vi "DSPS_E36000.Manager.vi"(11 "Module Config":T2={"Name"="Serial Port", "Parent Q"=refnum, "Is Child?"=FALSE, "Index"=0, "Dirs"={"Root"=path "", "Config"=path "C:/ATE/Config", "Logs"=path "C:/ATE/Logs", "Reports"=path "C:/ATE/Reports", "App Data"=path "C:/ProgramData/MAIN"}, "Simulate"=FALSE, "SimCtrl"=refnum}) -> ()   [LabVIEW 2018]
uses:
  <vilib>/KATE/Module/Module Config.ctl
  <vilib>/KATE/Queues/Q.Element.ctl
  <vilib>/KATE/Module/Module.Working Dirs.ctl
  <vilib>/KATE/Event Log/Event Notification/Event Log.Log Level.ctl
  <vilib>/KATE/Module/Module.SW Version Info.ctl
  <vilib>/KATE/Module/Window/Window.Task, Action.ctl
  Utils/Functions/FunctMgr/FunctMgr.lvclass
  Utils/Errors/Error.Error Code List.ctl
  <vilib>/Utility/sysdir.llb/System Directory Type.ctl
  <vilib>/KATE/Event Log/Event Notification/Event Log.Notification Type.ctl
  <vilib>/KATE/Config/Stored Controls/Class.SaveCtrls.lvclass
  <vilib>/KATE/Queues/Queue Utils.lvlib
  <vilib>/KATE/Module/Module Utils.lvlib
  <vilib>/KATE/Event Log/Event Log.lvlib
  <vilib>/KATE/Scheduler/Scheduler.lvlib
  <vilib>/KATE/Menu/Menu Utils.lvlib
  <vilib>/KATE/Config/Config Utils.lvlib
  <vilib>/KATE/Status/Status Utils.lvlib
  <vilib>/KATE/Files/File Utils.lvlib
  <vilib>/KATE/SeqMgr/SeqMgr.lvlib
  <vilib>/KATE/Event Log/Event Notification/Event Notification.lvclass
panel:
  in  "Main Tab":enum32{"Operate", "Maint"}(tab)
  in  "Data Tab":enum32{"Control", "Config"}(tab)
  in  "Save Current to File":bool
  out "PS Output State":bool
  in  "Interval(s)":dbl=0.1 min=0.1 max=10.0 step=0.1
  in  "Continuous Read":bool
  in  "Current Lim":dbl=1.0
  in  "PS - Set Output OFF":bool
  in  "Voltage":dbl=12.0
  out "Current(A)":dbl format="%#.3f"
  in  "Read Current":bool
  in  "PS - Set Output ON":bool
  in  "Alias":refnum<visa-resource-name>="PS1"
  out "Status":string
  out "Current Graph":cluster{"t":dbl[], "Y":dbl[]}(graph)
  in  "Clear Current Graph":bool
  out "CurrAvg(A)":dbl caption="Average(A)" format="%#.3f"
  out "CurrPeak(A)":dbl caption="Peak(A)" format="%#.3f"
  in  "Average Cnt":i32=1 caption="Average Samples" min=1 max=100 step=1
  in  "Toggle Sim":bool
  in  "Get ID":bool
  out "FW":string
  out "SN":string
  out "Model":string
  out "Mfg":string
  out "Error":errorcluster
  in  "Logging Level":T1
  out "Rev":string="v1.0.0"
  out "Simulate Indication":string="Simulating Instruments"
  out "Error Status":string
  in  "Clear Error":bool
  in  "Leave Maint":bool
  # "Power Supply Manager"
  # "Output"
  # "V"
  # "A"
  # "Current"
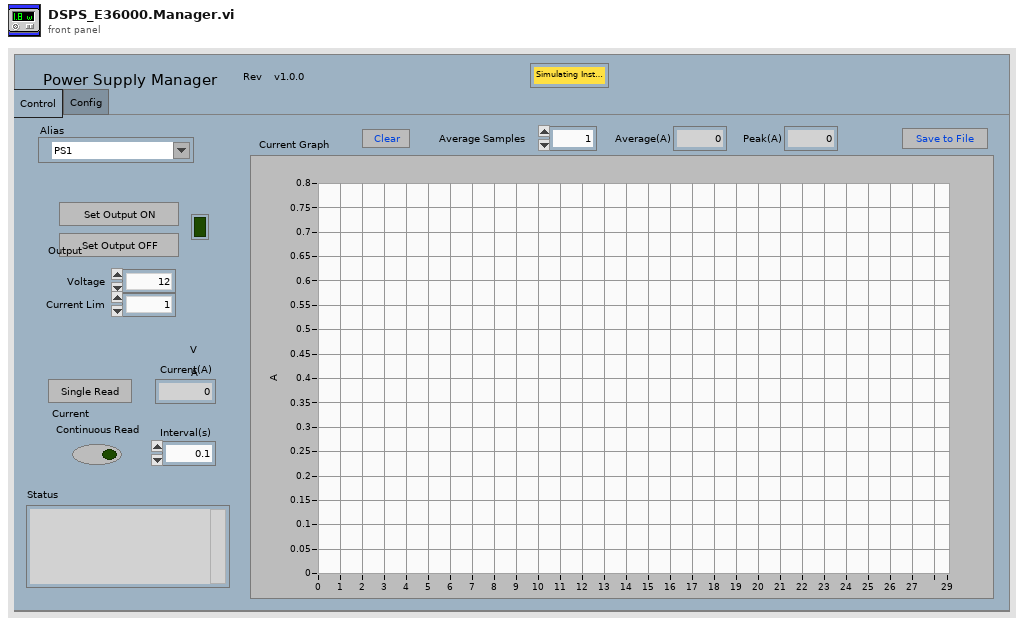
[diagram p1: front panel]
types:
  T1 = typedef "KATE_Lib.lvlib/Event Log.lvlib/Event Log.Log Level.ctl" = enum16{"Normal", "Verbose", "Debug0", "Debug1", "Debug2"}
  T2 = typedef "KATE_Lib.lvlib/Module Utils.lvlib/Module Config.ctl" = cluster{"Name":string, "Parent Q":refnum<queue>, "Is Child?":bool, "Index":i32, "Dirs":T3, "Simulate":bool, "SimCtrl":refnum<vi>}
  T3 = typedef "KATE_Lib.lvlib/Module Utils.lvlib/Module.Working Dirs.ctl" = cluster{"Root":path, "Config":path, "Logs":path, "Reports":path, "App Data":path}
  T4 = typedef "KATE_Lib.lvlib/Module Utils.lvlib/Module.SW Version Info.ctl" = cluster{"AppName":string, "Company":string, "Version":string, "Description":string, "PN":string}
  T5 = typedef "KATE_Lib.lvlib/Module Utils.lvlib/Module Sys Info.ctl" = cluster{"Main Q":refnum<queue>, "Exe":bool, "SW Rev":T4, "Self Ref":refnum<vi>, "Main Tab":refnum<vi>, "Pane":refnum<vi>, "Stop":cluster{"Ref":refnum<event-registration>, "Event":refnum<user-event>}, "Cfg":T2, "Services":cluster{"Name":string, "vi ref":refnum<vi>}[], "Menu Ref":refnum<k9>, "CtrlStates":refnum<class "Class.SaveCtrls.lvclass">, "Docs":cluster{"Tags":string[], "Paths":path[]}, "Log":refnum<class "Event Notification.lvclass">, "Test Controls":refnum<vi>[], "Child Modules":cluster{"Name":string, "vi ref":refnum<vi>}[], "SW Items":string[][], "AppData":refnum<class "Class.AppData.lvclass">}
  T6 = enum8{"Enabled", "Disabled", "Disabled and Grayed Out"}
  T7 = enum16{"open", "replace", "create", "open or create", "replace or create", "replace or create with confirmation"}
  T8 = typedef "KATE_Lib.lvlib/Event Log.lvlib/Event Log.Notification Type.ctl" = enum16{"Normal", "Warning", "Error", "Success"}
  T9 = cluster{"Child Modules":cluster{"VI Ref":refnum<vi>, "Name":string}[]}
  T10 = cluster{"Local Error":errorcluster, "Lnch":bool, "FunctMgr":refnum<class "FunctMgr.lvclass">, "App":cluster{"Child Modules":cluster{"VI Ref":refnum<vi>, "Name":string}[]}, "Alias":refnum<visa-resource-name>, "GraphData":cluster{"t":dbl[], "Y":dbl[]}, "Current":dbl, "GraphStart":dbl, "Connected":bool}
  T11 = typedef "Error.Error Code List.ctl" = i32
  T12 = typedef "System Directory Type.ctl" = i32
  T13 = typedef "KATE_Lib.lvlib/Module Utils.lvlib/Window.Task, Action.ctl" = enum16{"Resize()", "Show Panel(Bool)", "Show Scroll Bars(Bool)", "Dock to SubPanel(SubPanel Ref)", "Undock from SubPanel()", "Return to SubPanel()", "Go To Maint Tab()", "Show Maint Tab(Bool)", "Open Block Diagram()"}
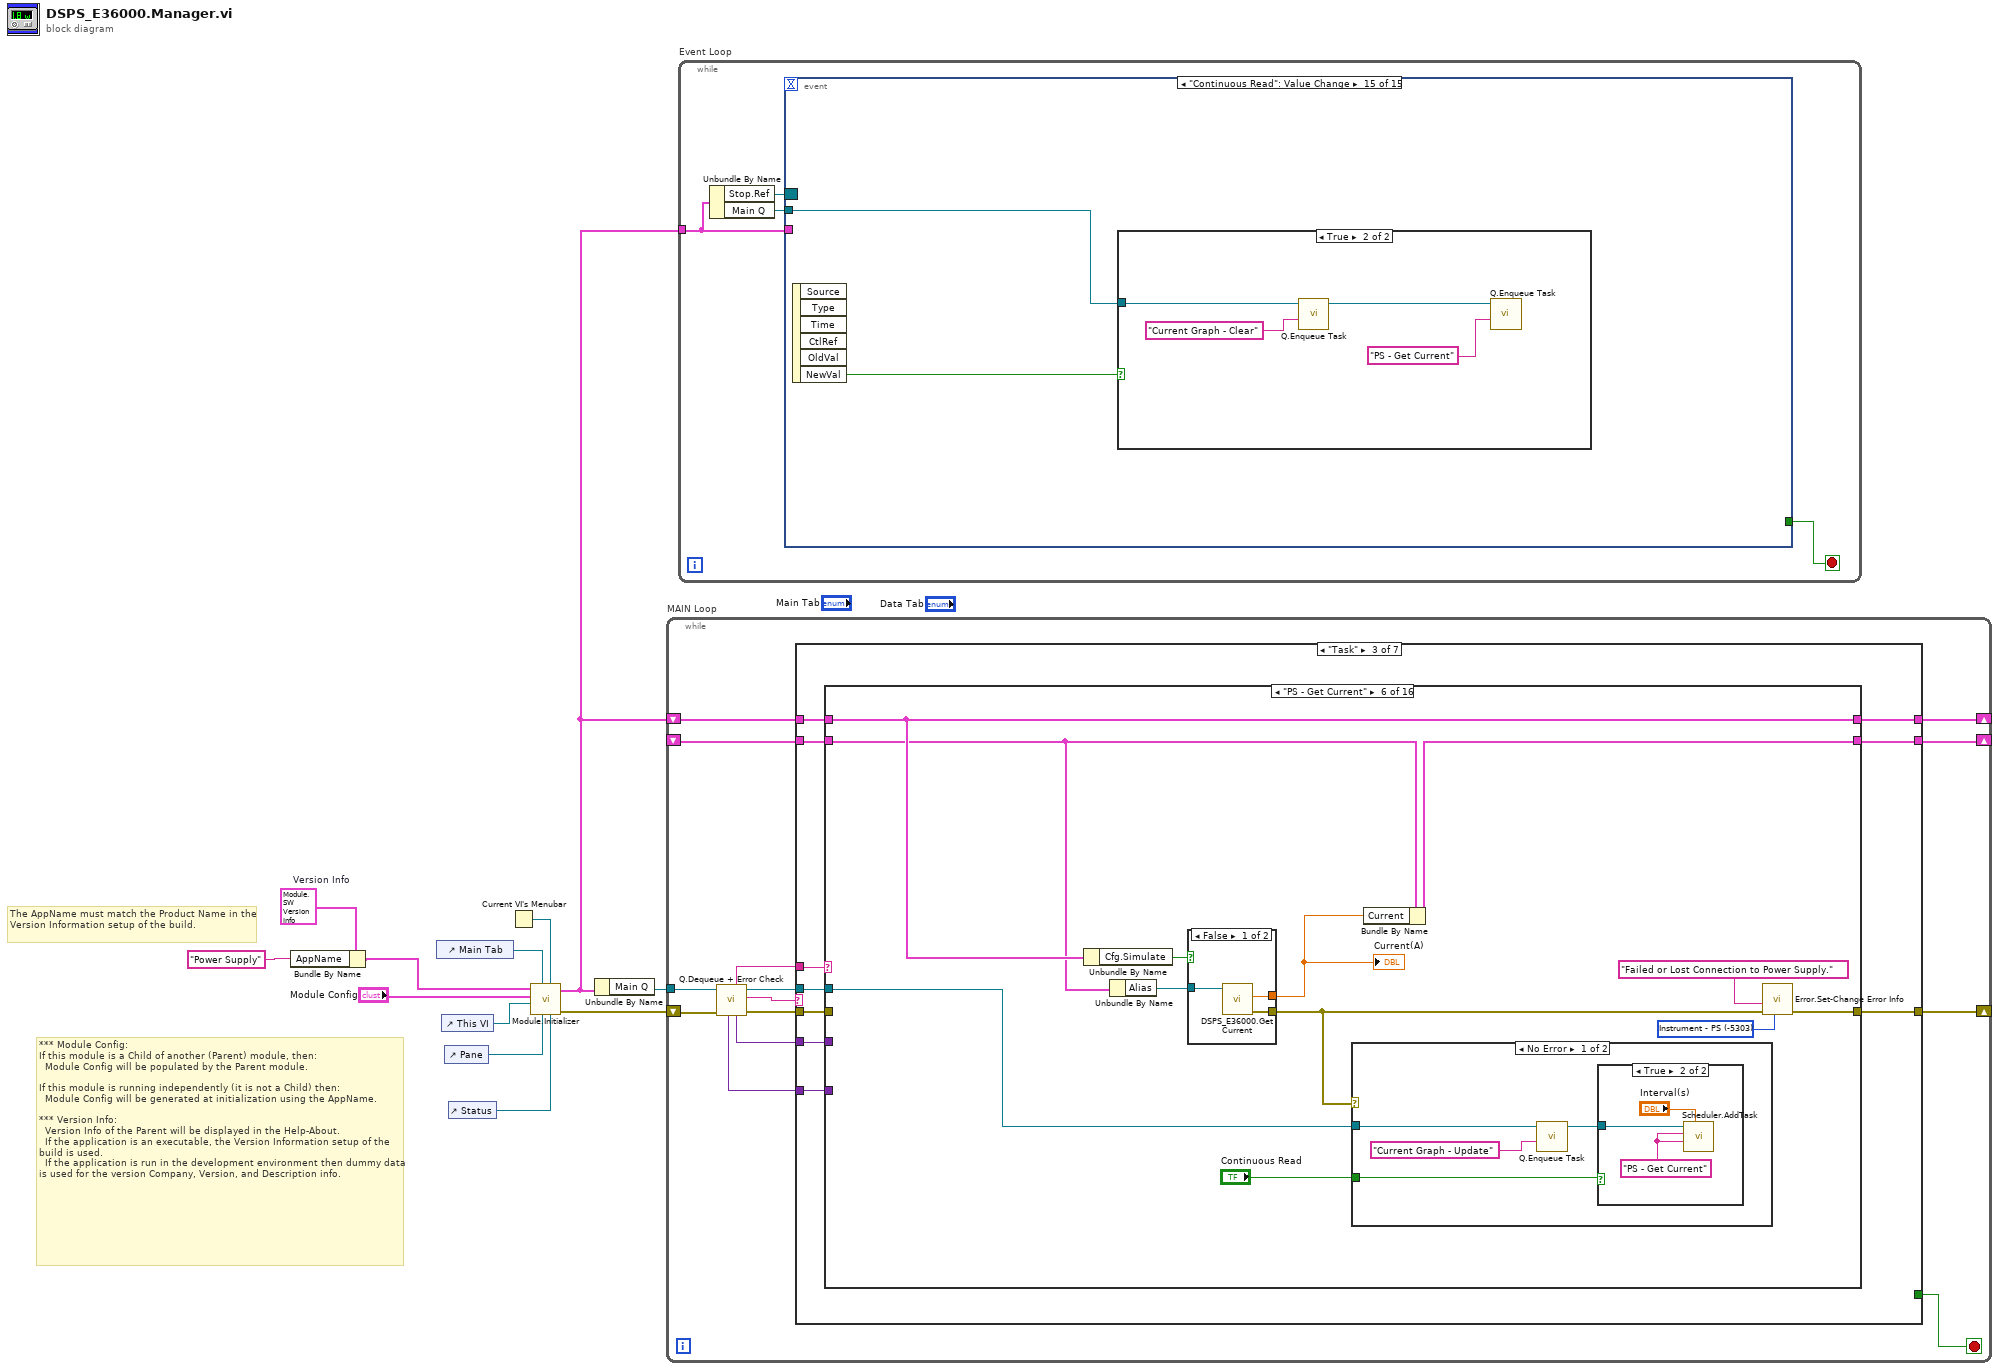
[diagram p0: block diagram]
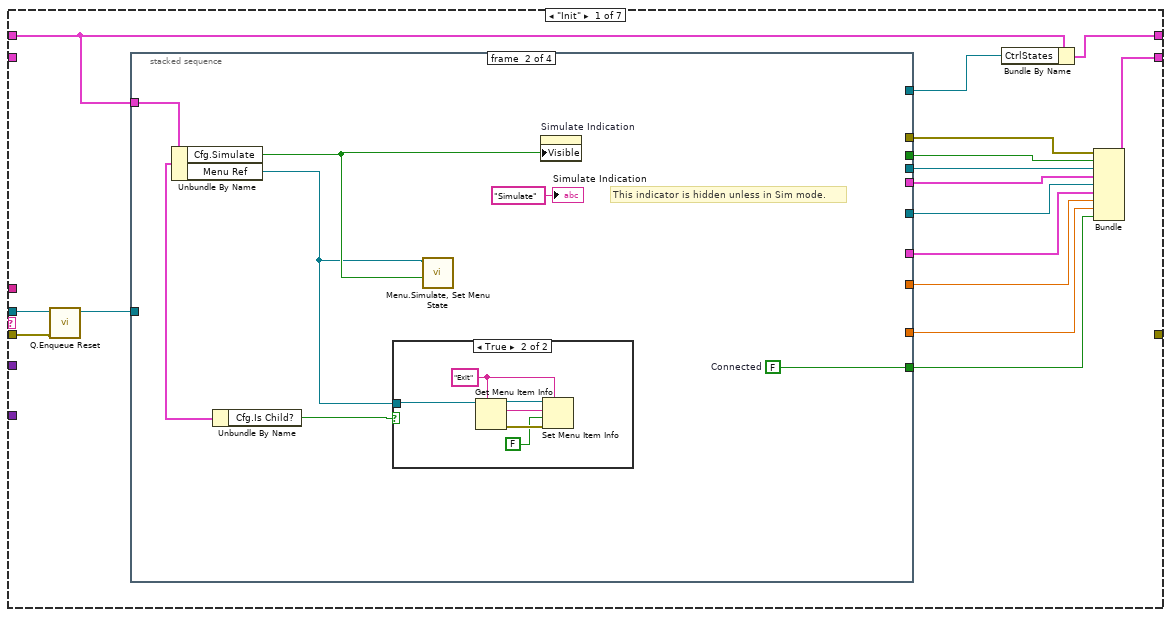
[diagram p2: hidden frame]
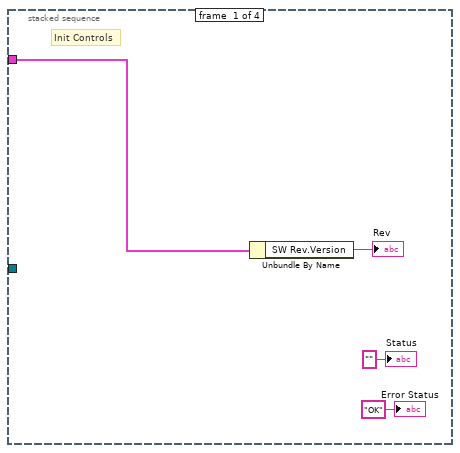
[diagram p3: hidden frame]
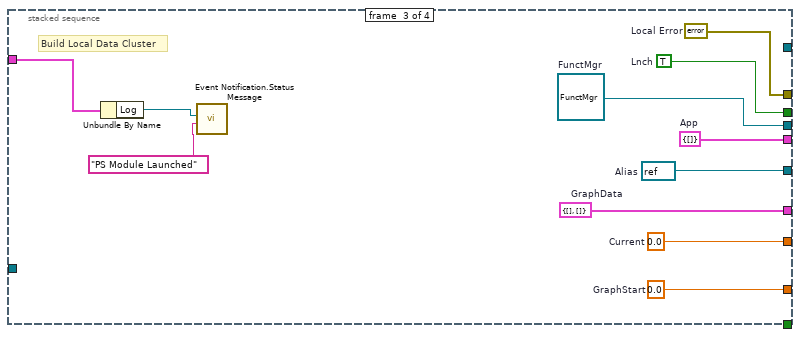
[diagram p5: hidden frame]
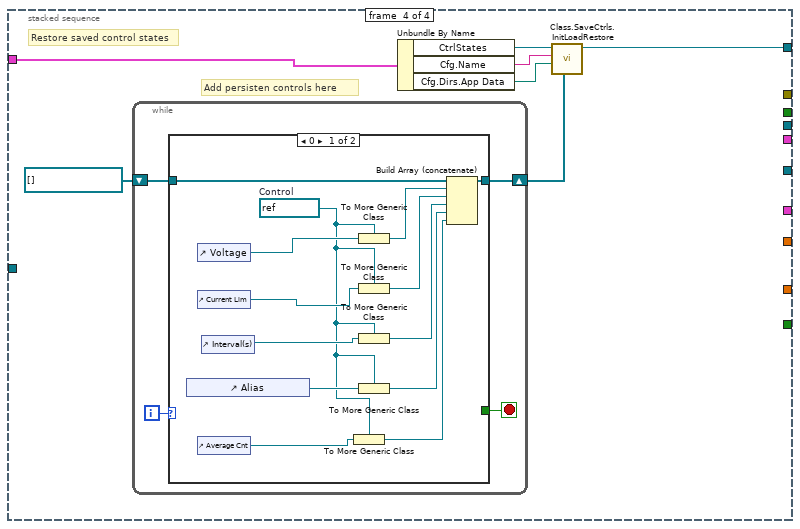
[diagram p6: hidden frame]
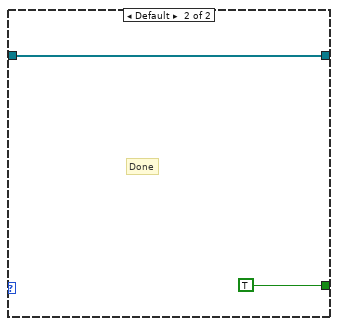
[diagram p7: hidden frame]
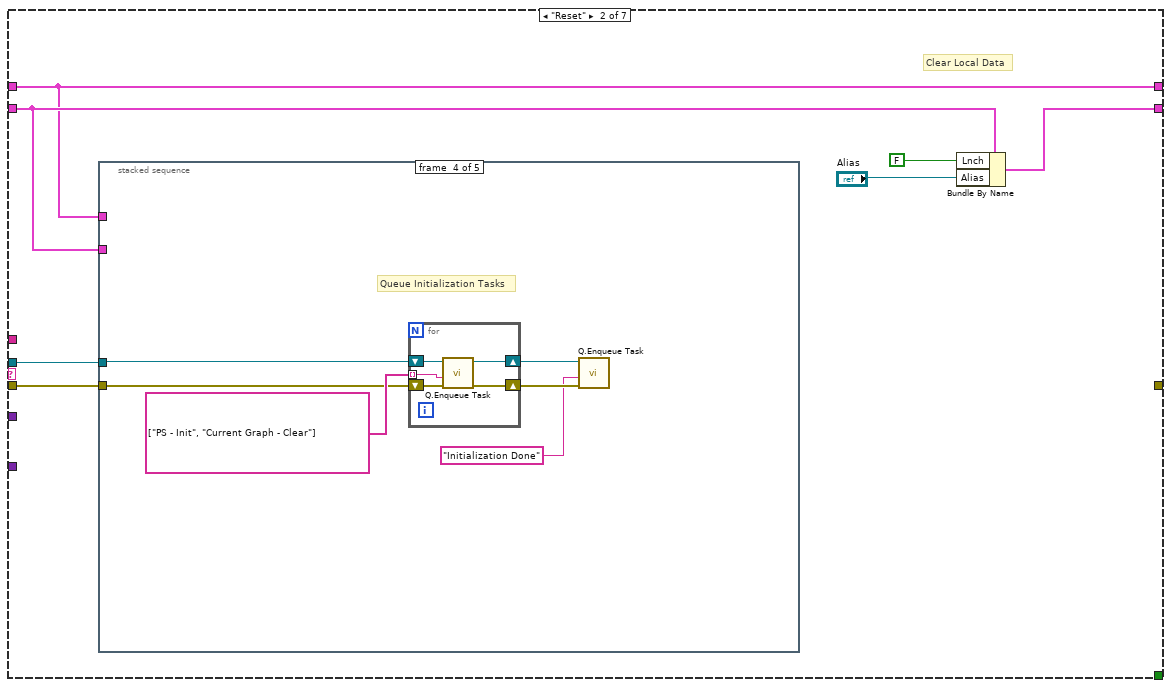
[diagram p8: hidden frame]
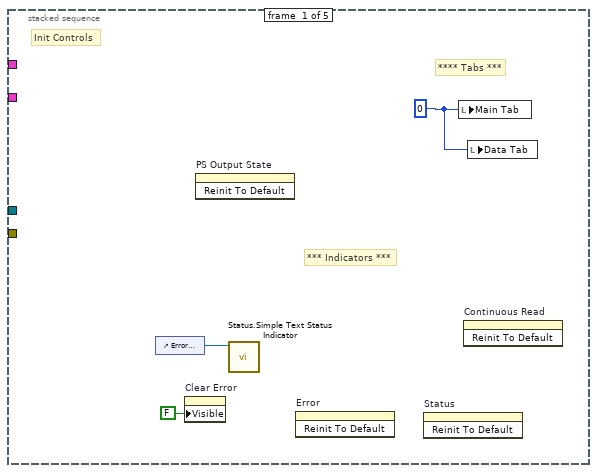
[diagram p9: hidden frame]
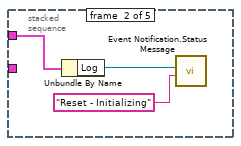
[diagram p10: hidden frame]
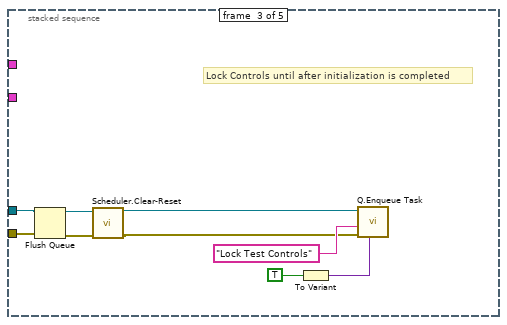
[diagram p11: hidden frame]
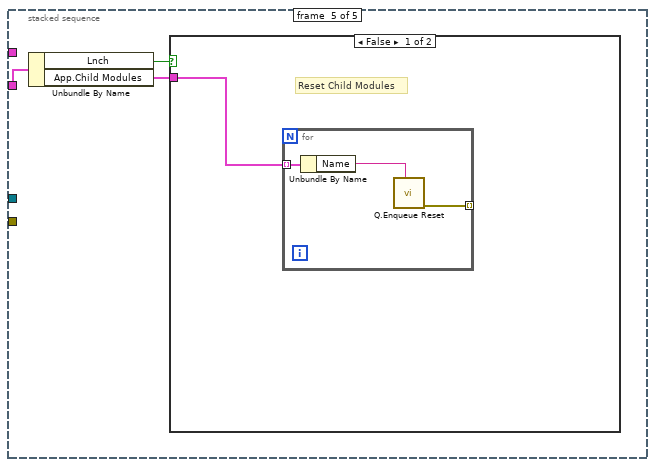
[diagram p12: hidden frame]
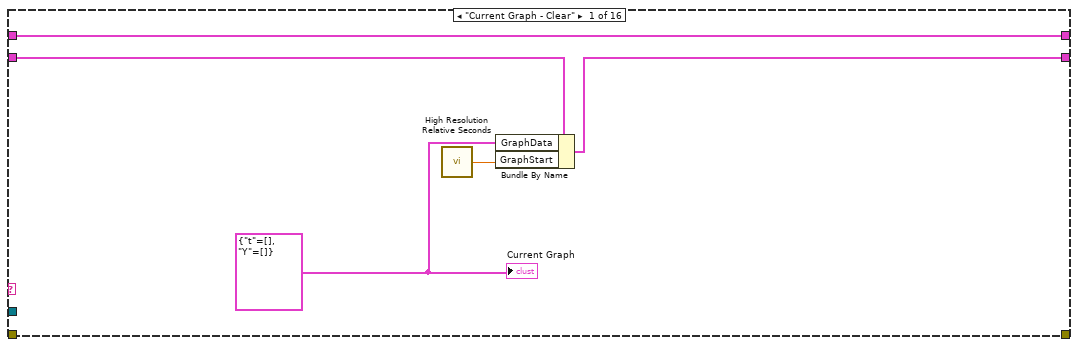
[diagram p14: hidden frame]
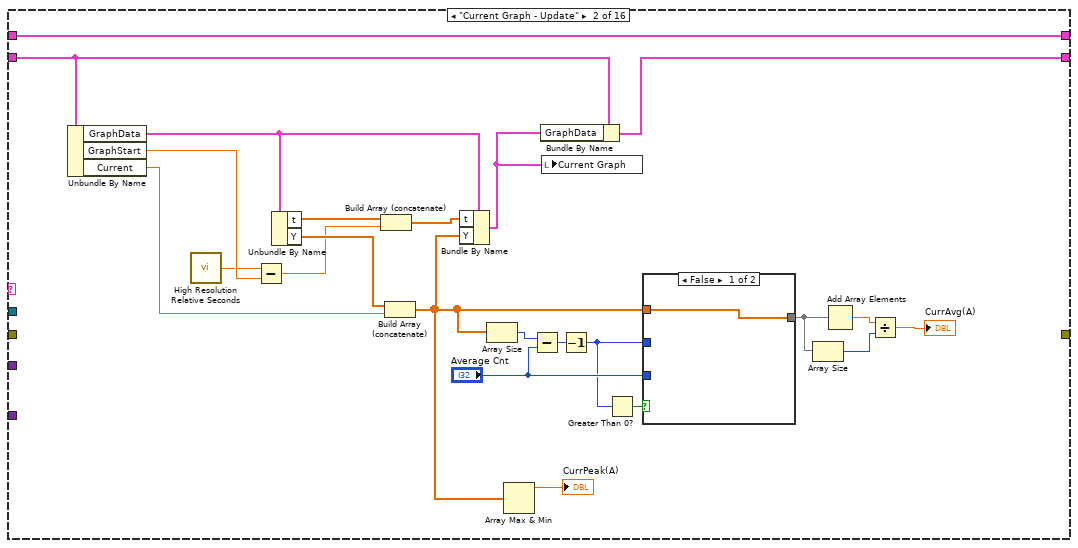
[diagram p15: hidden frame]
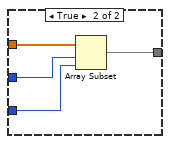
[diagram p16: hidden frame]
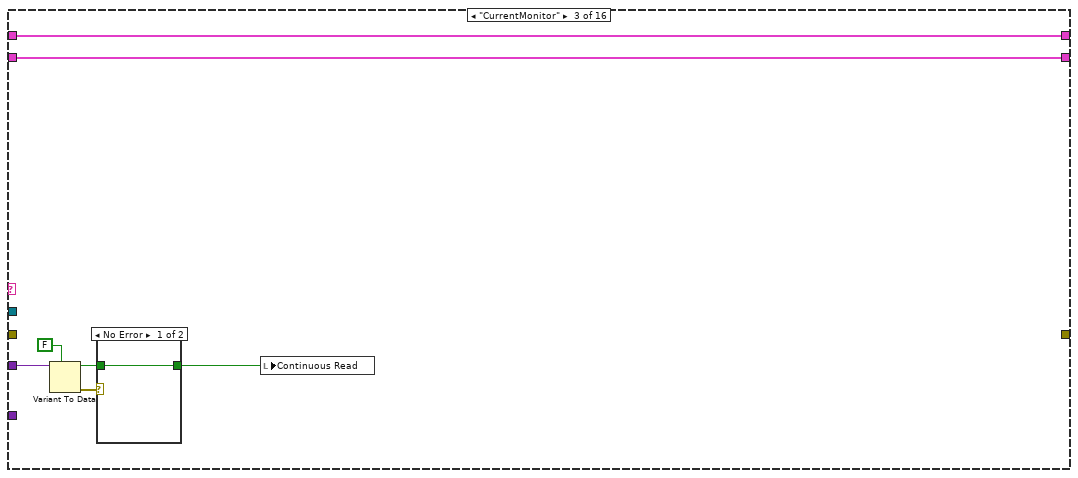
[diagram p17: hidden frame]
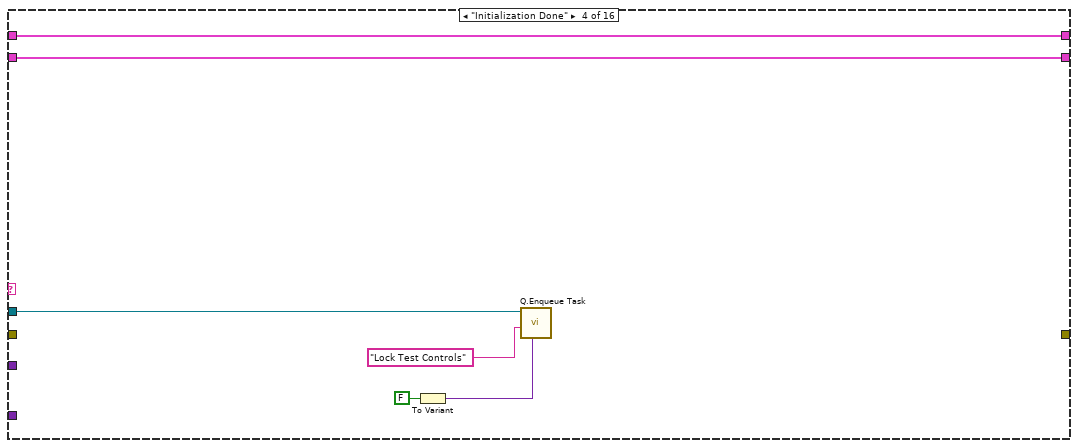
[diagram p19: hidden frame]
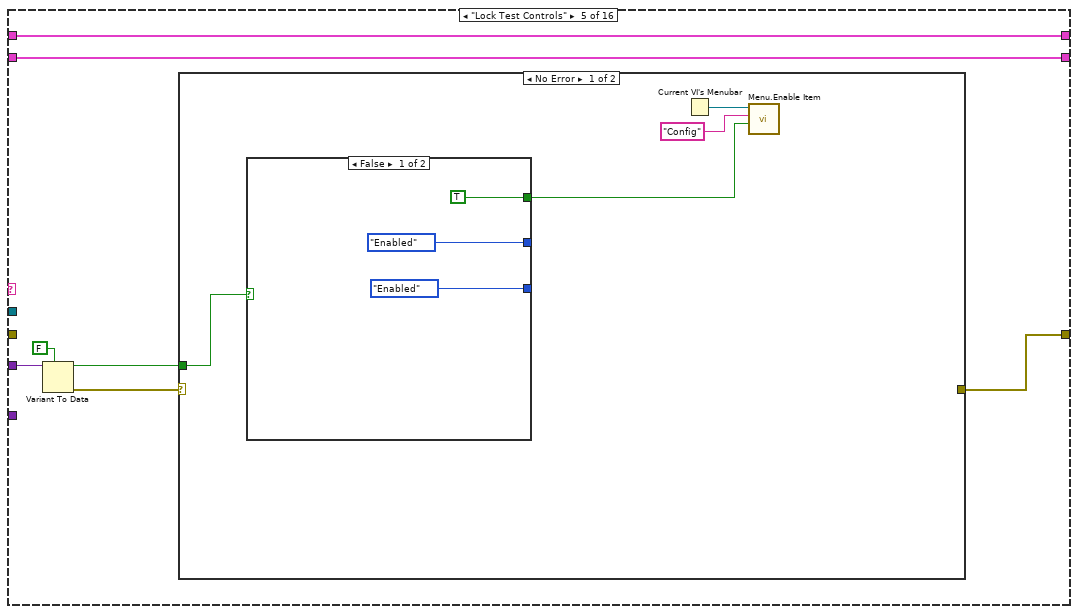
[diagram p20: hidden frame]
diagram:
  w2 = T4 {"AppName"="ModuleX", "Company"="CompanyX", "Version"="1.0", "Description"="This app is being developed.", "PN"=""}  # Version Info
  # "*** Module Config:\nIf this module is a Child of another (Parent) module, then:\n  Module Config will be populated by the Parent module.\n\nIf this module is running independently (it is not a Child) then:\n  Module Config will be generated at initialization using the AppName.\n\n*** Version Info:\n  Version Info of the Parent will be displayed in the Help-About.\n  If the application is an executable, the Version Information setup of the build is used.\n  If the application is run in the development environment then dummy data is used for the version Company, Version, and Description info."
  # "The AppName must match the Product Name in the Version Information setup of the build."
  n1 = Bundle By Name(cluster=w2, "AppName"="Power Supply") -> (w1:T4)
  n2 = control-ref of="Main Tab"() -> (w10:refnum<vi>)
  n3 = control-ref of="This VI"() -> (w9:refnum<vi>)
  n4 = control-ref of="Pane"() -> (w8:refnum<vi>)
  n5 = control-ref of="Status"() -> (w4:refnum<vi>)
  n6 = Current VI's Menubar() -> (w6:refnum<k9>)
  n7 = call <vilib>:"Module.Initializer.vi"("StatusTxtBx"=w4, "Menu Ref"=w6, "Pane"=w8, "Main Tab"=w10, "Self Ref"=w9, "Module Config"="Module Config", "SW Rev"=w1) -> ("error out"=w12:errorcluster, "Sys"=w7:T5)  [unwired: 3 in]
  n8 = Unbundle By Name(w7) -> ("Main Q"=w11:refnum<queue>)
  n9 = while "MAIN Loop" {
    shift-right: [w23] -> _
    shift-left: w12 -> [w21]
    shift-right: [w24] -> _
    shift-left: _ -> [w13]
    shift-right: [w25] -> _
    shift-left: w7 -> [w26]
    tunnel: w11 -> [w20]
    stop <- w15 stop-if-true
    n10 = call <vilib>:"Q.Dequeue + Error Check.vi"("Error In"=w21, "Q In"=w20) -> ("error out"=w22:errorcluster, "Cmd"=w19:string, "Q Out"=w18:refnum<queue>, "Data1"=w17:variant, "Sub"=w14:string, "Data2"=w16:variant)  [unwired: 4 in]
    n11 = case shown="\"Task\"" w19 {
      selector: w19 -> [_ _ _ _ _ w612 _]
      tunnel: w13 -> [_ w99 w144 w407 w586 w606 w671]
      tunnel: w26 -> [w37 w97 w145 w408 w587 w607 w672]
      tunnel: [w38 w97 w143 w406 w585 w607 w672] -> w25
      tunnel: [w40 w102 w142 w405 w584 w605 w671] -> w24
      tunnel: [_ _ w136 w400 _ w613 w674] -> w23
      tunnel: w22 -> [w41 w100 w138 w401 _ w610 _]
      tunnel: w18 -> [w42 w101 w139 w402 w590 w608 _]
      tunnel: w17 -> [_ _ w140 w403 w589 w611 _]
      tunnel: w16 -> [_ _ w137 w399 w588 _ _]
      tunnel: w14 -> [_ _ w141 w404 w591 w609 _]
      tunnel: [_ _ _ _ _ _ TRUE] -> w15
      frame "Init" {
        n12 = call <vilib>:"Q.Enqueue Reset.vi"("Error In"=w41, "Q In"=w42) -> ("Q Out"=w35:refnum<queue>)  [unwired: 8 in, 1 out]
        n13 = stacked-sequence {
          tunnel: [_ _ w63 _] -> w39
          tunnel: w37 -> [w45 w49 w66 w71]
          tunnel: [_ _ _ w70] -> w36
          tunnel: w35 -> [_ _ _ _]
          tunnel: [_ _ w69 _] -> w34
          tunnel: [_ _ w68 _] -> w33
          tunnel: [_ _ w61 _] -> w32
          tunnel: [_ _ w67 _] -> w31
          tunnel: [_ _ w62 _] -> w30
          tunnel: [_ _ w60 _] -> w29
          tunnel: [_ _ w59 _] -> w28
          tunnel: [_ w47 _ _] -> w27
          frame #0 {
            # "Init Controls"
            n14 = Unbundle By Name(w45) -> ("SW Rev.Version"=→"Rev":string)
            "Status" <- "" ("Status")
            "Error Status" <- "OK" ("Error Status")
          }
          frame #1 {
            w47 = FALSE  # Connected
            # "This indicator is hidden unless in Sim mode."
            n15 = Unbundle By Name(w49) -> ("Cfg.Simulate"=w51:bool, "Menu Ref"=w48:refnum<k9>)
            n16 = Unbundle By Name(w49) -> ("Cfg.Is Child?"=w50:bool)
            n17 = case shown="True" w50 {
              tunnel: w48 -> [_ w54]
              frame False {
              }
              frame True {
                w56 = "Exit"
                n18 = Get Menu Item Info(7:w56, 11:w54) -> (0:w55:errorcluster, 2:w57:string, 3:w58:refnum<k9>)  [unwired: 1 in, 4 out]
                n19 = Set Menu Item Info(7:w56, 8:w55, 9:FALSE ("enabled"), 10:w57, 11:w58) -> ()  [unwired: 2 in, 2 out]
              }
            }
            n20 = call <vilib>:"Menu.Simulate, Set Menu State.vi"("Sim Enable"=w51, "Menu Ref"=w48) -> ()  [unwired: 8 in, 2 out]
            n21 = property on="Simulate Indication" class="Str"("Visible"=w51) -> ()  [unwired: 2 in, 2 out]
            "Simulate Indication" <- "Simulate" ("Simulate Indication")
          }
          frame #2 {
            w59 = 0.0  # GraphStart
            w60 = 0.0  # Current
            w61 = refnum<visa-resource-name> refnum  # Alias
            w62 = cluster{"t":dbl[], "Y":dbl[]} {"t"=[], "Y"=[]}  # GraphData
            w67 = errorcluster {"status"=FALSE, "code"=0, "source"=""}  # Local Error
            w63 = refnum<class "FunctMgr.lvclass"> refnum  # FunctMgr
            w68 = T9 {"Child Modules"=[]}  # App
            w69 = TRUE  # Lnch
            # "Build Local Data Cluster"
            n22 = Unbundle By Name(w66) -> ("Log"=w65:refnum<class "Event Notification.lvclass">)
            n23 = call <vilib>:"Event Notification.Status Message.vi"("Message"="PS Module Launched", "Event Notification in"=w65) -> ()  [unwired: 10 in]
          }
          frame #3 {
            # "Add persisten controls here"
            # "Restore saved control states"
            n24 = while {
              shift-right: [w78] -> w72
              shift-left: refnum<vi>[] [] -> [w79]
              i -> [w80]
              stop <- w77 stop-if-true
              n25 = case shown="0" w80 {
                tunnel: w79 -> [w92 w95]
                tunnel: [w93 w95] -> w78
                tunnel: [_ TRUE] -> w77
                frame 0 {
                  w83 = refnum<vi> refnum  # Control
                  n26 = control-ref of="Alias"() -> (w87:refnum<vi>)
                  n27 = control-ref of="Voltage"() -> (w84:refnum<vi>)
                  n28 = control-ref of="Current Lim"() -> (w85:refnum<vi>)
                  n29 = control-ref of="Average Cnt"() -> (w81:refnum<vi>)
                  n30 = control-ref of="Interval(s)"() -> (w86:refnum<vi>)
                  n31 = To More Generic Class(target class=w83, reference=w81) -> (generic class reference=w82:refnum<vi>)
                  n32 = To More Generic Class(target class=w83, reference=w84) -> (generic class reference=w91:refnum<vi>)
                  n33 = To More Generic Class(target class=w83, reference=w85) -> (generic class reference=w90:refnum<vi>)
                  n34 = To More Generic Class(target class=w83, reference=w86) -> (generic class reference=w89:refnum<vi>)
                  n35 = To More Generic Class(target class=w83, reference=w87) -> (generic class reference=w88:refnum<vi>)
                  n36 = Build Array (concatenate)(w92, w91, w90, w89, w88, w82) -> (w93:refnum<vi>[])
                }
                frame Default {
                  # "Done"
                }
              }
            }
            n37 = Unbundle By Name(w71) -> ("CtrlStates"=w73:refnum<class "Class.SaveCtrls.lvclass">, "Cfg.Name"=w75:string, "Cfg.Dirs.App Data"=w74:path)
            n38 = call-dynamic "Class.SaveCtrls.InitLoadRestore.vi"("Ctrl Array"=w72, "Module Data Dir"=w74, "Module Name"=w75, "CtrlStates In"=w73) -> ("CtrlStates"=w70:refnum<class "Class.SaveCtrls.lvclass">)  [unwired: 6 in, 1 out]
          }
        }
        n39 = Bundle By Name(cluster=w37, "CtrlStates"=w36) -> (w38:T5)
        n40 = Bundle("Local Error"=w31, "Lnch"=w34, "FunctMgr"=w39, "App"=w33, "Alias"=w32, "GraphData"=w30, "Current"=w29, "GraphStart"=w28, "Connected"=w27) -> (w40:T10)  [unwired: 1 in]
      }
      frame "Reset" {
        # "Clear Local Data"
        n41 = stacked-sequence {
          tunnel: w101 -> [_ _ w110 w118 _]
          tunnel: w100 -> [_ _ w109 w122 _]
          tunnel: w99 -> [_ _ _ _ w131]
          tunnel: w97 -> [_ w108 _ _ _]
          frame #0 {
            w105 = 0
            # "*** Indicators ***"
            # "**** Tabs ***"
            # "Init Controls"
            n42 = control-ref of="Error Status"() -> (w104:refnum<vi>)
            n43 = property on="Clear Error" class="Bool"("Visible"=FALSE) -> ()  [unwired: 2 in, 2 out]
            n44 = invoke on="PS Output State" class="Bool (strict)" method="Reinit To Default"() -> ()  [unwired: 3 in, 3 out]
            n45 = call <vilib>:"Status.Simple Text Status Indicator.vi"("Status TextBox"=w104) -> ()  [unwired: 10 in, 1 out]
            n46 = invoke on="Error" class="Clust (strict)" method="Reinit To Default"() -> ()  [unwired: 3 in, 3 out]
            n47 = invoke on="Status" class="Str" method="Reinit To Default"() -> ()  [unwired: 3 in, 3 out]
            n48 = local write "Main Tab"(w105) -> ()
            n49 = invoke on="Continuous Read" class="Bool (strict)" method="Reinit To Default"() -> ()  [unwired: 3 in, 3 out]
            n50 = local write "Data Tab"(w105) -> ()
          }
          frame #1 {
            n51 = Unbundle By Name(w108) -> ("Log"=w107:refnum<class "Event Notification.lvclass">)
            n52 = call <vilib>:"Event Notification.Status Message.vi"("Message"="Reset - Initializing", "Event Notification in"=w107) -> ()  [unwired: 10 in]
          }
          frame #2 {
            # "Lock Controls until after initialization is completed"
            n53 = Flush Queue(queue=w110, error in (no error)=w109) -> (queue out=w111:refnum<queue>, error out=w114:errorcluster)  [unwired: 1 out]
            n54 = call <vilib>:"Scheduler.Clear-Reset.vi"("error in"=w114, "Q In"=w111) -> ("error out"=w112:errorcluster, "Q Out"=w113:refnum<queue>)  [unwired: 8 in]
            n55 = To Variant(anything=TRUE) -> (Variant=w116:variant)
            n56 = call <vilib>:"Q.Enqueue Task.vi"("Data1"=w116, "Error In"=w112, "Task Name"="Lock Test Controls", "Q In"=w113) -> ()  [unwired: 6 in, 2 out]
          }
          frame #3 {
            # "Queue Initialization Tasks"
            n57 = for {
              shift-right: [w126] -> w120
              shift-left: w122 -> [w127]
              tunnel: string[] ["PS - Init", "Current Graph - Clear"] -> [w124] mode=indexing
              shift-right: [w125] -> w121
              shift-left: w118 -> [w128]
              n58 = call <vilib>:"Q.Enqueue Task.vi"("Error In"=w127, "Task Name"=w124, "Q In"=w128) -> ("error out"=w126:errorcluster, "Q Out"=w125:refnum<queue>)  [unwired: 7 in]
            }
            n59 = call <vilib>:"Q.Enqueue Task.vi"("Error In"=w120, "Task Name"="Initialization Done", "Q In"=w121) -> ()  [unwired: 7 in, 2 out]
          }
          frame #4 {
            n60 = Unbundle By Name(w131) -> ("Lnch"=w130:bool, "App.Child Modules"=w129:cluster{"VI Ref":refnum<vi>, "Name":string}[])
            n61 = case shown="False" w130 {
              tunnel: w129 -> [w132 _]
              frame False {
                # "Reset Child Modules"
                n62 = for {
                  tunnel: w132 -> [w135] mode=indexing
                  tunnel: [w133] -> _ mode=indexing
                  n63 = Unbundle By Name(w135) -> ("Name"=w134:string)
                  n64 = call <vilib>:"Q.Enqueue Reset.vi"("Q Name"=w134) -> ("error out"=w133:errorcluster)  [unwired: 9 in, 1 out]
                }
              }
              frame True {
                # "Do not reset at launch.\nThey are already reset"
              }
            }
          }
        }
        n65 = Bundle By Name(cluster=w99, "Lnch"=FALSE ("Test.Running"), "Alias"="Alias") -> (w102:T10)
      }
      frame "Task" {
        n66 = case shown="\"PS - Get Current\"" w141 {
          selector: w141 -> [_ _ _ _ _ _ _ _ _ _ _ _ _ _ _ w394]
          tunnel: w145 -> [w150 w173 w185 w192 w199 w220 w241 w265 w291 w309 w345 w351 w356 w372 w378 w389]
          tunnel: w144 -> [w149 w168 w184 w187 w193 w217 w247 w260 w293 w305 w344 w350 w360 w374 w377 w395]
          tunnel: [w150 w173 w185 w192 w199 w220 w241 w265 w291 w309 w345 w351 w361 w373 w378 w388] -> w143
          tunnel: [w148 w167 w184 w187 w193 w216 w247 w259 w293 w304 w344 w349 w360 w374 w377 w395] -> w142
          tunnel: w140 -> [_ _ w183 _ w198 _ _ _ w289 w301 _ _ w363 _ w379 w393]
          tunnel: w139 -> [_ _ _ w191 _ w221 _ w266 _ _ _ _ w357 w375 _ _]
          tunnel: w138 -> [_ _ _ _ _ _ _ _ _ _ _ _ _ _ _ w391]
          tunnel: w137 -> [_ _ _ _ _ _ _ _ _ w302 _ _ _ _ _ w392]
          tunnel: [_ _ _ _ w195 w212 w237 w256 w284 w303 _ _ _ _ w376 w390] -> w136
          frame "Current Graph - Clear" {
            w147 = cluster{"t":dbl[], "Y":dbl[]} {"t"=[], "Y"=[]}
            n67 = call <vilib>:"High Resolution Relative Seconds.vi"() -> ("relative seconds"=w146:dbl)
            n68 = Bundle By Name(cluster=w149, "GraphData"=w147, "GraphStart"=w146) -> (w148:T10)
            "Current Graph" <- w147
          }
          frame "Current Graph - Update" {
            n69 = Unbundle By Name(w168) -> ("GraphData"=w169:cluster{"t":dbl[], "Y":dbl[]}, "GraphStart"=w154:dbl, "Current"=w151:dbl)
            n70 = call <vilib>:"High Resolution Relative Seconds.vi"() -> ("relative seconds"=w153:dbl)
            n71 = Subtract(x=w153, y=w154) -> (x-y=w152:dbl)
            n72 = Unbundle By Name(w169) -> ("t"=w172:dbl[], "Y"=w170:dbl[])
            n73 = Build Array (concatenate)(w172, w152) -> (w171:dbl[])
            n74 = Build Array (concatenate)(w170, w151) -> (w165:dbl[])
            n75 = Bundle By Name(cluster=w169, "t"=w171, "Y"=w165) -> (w156:cluster{"t":dbl[], "Y":dbl[]})
            n76 = Array Size(array=w165) -> (size(s)=w164:i32)
            n77 = Array Max & Min(array=w165) -> (max value=→"CurrPeak(A)":dbl)  [unwired: 3 out]
            n78 = Subtract(x=w164, y="Average Cnt") -> (x-y=w163:i32)
            n79 = Bundle By Name(cluster=w168, "GraphData"=w156) -> (w167:T10)
            n80 = local write "Current Graph"(w156) -> ()
            n81 = Decrement(x=w163) -> (x-1=w160:i32)
            n82 = Greater Than 0?(x=w160) -> (x > 0?=w161:bool)
            n83 = case shown="False" w161 {
              tunnel: w165 -> [w174 w178]
              tunnel: w160 -> [_ w177]
              tunnel: "Average Cnt" -> [_ w176]
              tunnel: [w174 w175] -> w159
              frame False {
              }
              frame True {
                n84 = Array Subset(array=w178, index=w177, length=w176) -> (w175:dbl[])
              }
            }
            n85 = Array Size(array=w159) -> (size(s)=w157:i32)
            n86 = Add Array Elements(numeric array=w159) -> (sum=w158:dbl)
            n87 = Divide(x=w158, y=w157) -> (x/y=→"CurrAvg(A)":dbl)
          }
          frame "CurrentMonitor" {
            n88 = Variant To Data(type=FALSE, Variant=w183) -> (data=w180:bool, error out=w181:errorcluster)  [unwired: 1 in]
            n89 = case shown="No Error" w181 {
              tunnel: w180 -> [w186 _]
              tunnel: [w186 _] -> w179
              frame No Error {
              }
              frame Error {
              }
            }
            n90 = local write "Continuous Read"(w179) -> ()
          }
          frame "Initialization Done" {
            n91 = To Variant(anything=FALSE) -> (Variant=w189:variant)
            n92 = call <vilib>:"Q.Enqueue Task.vi"("Data1"=w189, "Task Name"="Lock Test Controls", "Q In"=w191) -> ()  [unwired: 7 in, 2 out]
          }
          frame "Lock Test Controls" {
            n93 = Variant To Data(type=FALSE, Variant=w198) -> (data=w194:bool, error out=w196:errorcluster)  [unwired: 1 in]
            n94 = case shown="No Error" w196 {
              selector: w196 -> [_ w210]
              tunnel: w194 -> [w203 _]
              tunnel: [_ w210] -> w195
              frame No Error {
                n95 = case shown="False" w203 {
                  tunnel: [T6."Enabled" ("Disabled") T6."Disabled and Grayed Out" ("Disabled")] -> _
                  tunnel: [T6."Enabled" ("Disabled") T6."Disabled" ("Disabled")] -> _
                  tunnel: [TRUE ("Enable") FALSE ("Enable")] -> w200
                  frame False {
                  }
                  frame True {
                  }
                }
                n96 = Current VI's Menubar() -> (w201:refnum<k9>)
                n97 = call <vilib>:"Menu.Enable Item.vi"("Enable"=w200, "Tag"="Config", "Menu Ref"=w201) -> ()  [unwired: 7 in, 2 out]
              }
              frame Error {
              }
            }
          }
          frame "PS - Get Current" {
            w214 = T11 -5303 items=["No Error"=0, "Abort"=-2, "Misc"=-5000, "Fixture Error"=-5100, "File IO - General"=-5200, "FIle IO - Config Error"=-5201, "Instrument - General"=-5300, "Instrument - Serial Com"=-5301, "Instrument - Camera"=-5302, "Instrument - PS"=-5303, "Instrument - Oscilloscope"=-5304, "Instrument - Function Gen"=-5305, "Instrument - Load"=-5306, "Instrument - Meter"=-5307, "Instrument - Power Control"=-5308, "Instrument - Motion"=-5309, "Instrument - RF"=-5310, "System Exe"=-5400, "Image Processing"=-5500, "Communication"=-5600, "Script - Syntax Error"=-6000, "Script - Invalid Name or Param"=-6100, "Script - Timeout"=-6200, "Invalid Data"=-6300] ("Std Code")
            n98 = Unbundle By Name(w220) -> ("Cfg.Simulate"=w219:bool)
            n99 = Unbundle By Name(w217) -> ("Alias"=w222:refnum<visa-resource-name>)
            n100 = case shown="False" w219 {
              tunnel: w222 -> [w225 _]
              tunnel: [w224 w228] -> w215
              tunnel: [w223 _] -> w211
              frame False {
                n101 = call "DSPS_E36000.Get Current.vi"("VISA Alias"=w225) -> ("error out"=w223:errorcluster, "Current"=w224:dbl)  [unwired: 7 in, 2 out]
              }
              frame True {
                n102 = Random Number (0-1)() -> (number: 0 to 1=w227:dbl)
                n103 = Multiply(x=w227, y=0.8) -> (x*y=w228:dbl)
              }
            }
            "Current(A)" <- w215
            n104 = case shown="No Error" w211 {
              tunnel: w221 -> [w231 _]
              tunnel: "Continuous Read" -> [w229 _]
              frame No Error {
                n105 = call <vilib>:"Q.Enqueue Task.vi"("Task Name"="Current Graph - Update" ("Name"), "Q In"=w231) -> ("Q Out"=w230:refnum<queue>)  [unwired: 8 in, 1 out]
                n106 = case shown="True" w229 {
                  tunnel: w230 -> [_ w235]
                  frame False {
                  }
                  frame True {
                    w234 = "PS - Get Current" ("Name")
                    n107 = call <vilib>:"Scheduler.AddTask.vi"("Interval(s)"="Interval(s)", "Task Name"=w234, "Sched Name"=w234, "Q In"=w235) -> ()  [unwired: 6 in, 2 out]
                  }
                }
              }
              frame Error {
              }
            }
            n108 = Bundle By Name(cluster=w217, "Current"=w215) -> (w216:T10)
            n109 = call "Error.Set-Change Error Info.vi"("Std Code"=w214, "error in"=w211, "Description"="Failed or Lost Connection to Power Supply.") -> ("error out"=w212:errorcluster)  [unwired: 8 in]
          }
          frame "PS - Get ID" {
            w239 = T11 -5303 items=["No Error"=0, "Abort"=-2, "Misc"=-5000, "Fixture Error"=-5100, "File IO - General"=-5200, "FIle IO - Config Error"=-5201, "Instrument - General"=-5300, "Instrument - Serial Com"=-5301, "Instrument - Camera"=-5302, "Instrument - PS"=-5303, "Instrument - Oscilloscope"=-5304, "Instrument - Function Gen"=-5305, "Instrument - Load"=-5306, "Instrument - Meter"=-5307, "Instrument - Power Control"=-5308, "Instrument - Motion"=-5309, "Instrument - RF"=-5310, "System Exe"=-5400, "Image Processing"=-5500, "Communication"=-5600, "Script - Syntax Error"=-6000, "Script - Invalid Name or Param"=-6100, "Script - Timeout"=-6200, "Invalid Data"=-6300] ("Std Code")
            n110 = Unbundle By Name(w241) -> ("Cfg.Simulate"=w240:bool)
            n111 = Unbundle By Name(w247) -> ("Alias"=w246:refnum<visa-resource-name>)
            n112 = case shown="False" w240 {
              tunnel: w246 -> [w253 _]
              tunnel: [w252 _] -> w236
              tunnel: [w251 w254] -> w245
              tunnel: [w250 w254] -> w244
              tunnel: [w249 w254] -> w243
              tunnel: [w248 w254] -> w242
              frame False {
                n113 = call "DSPS_E36000.Get ID.vi"("VISA Alias"=w253) -> ("error out"=w252:errorcluster, "SN"=w250:string, "Model"=w249:string, "FW"=w251:string, "Mfg"=w248:string)  [unwired: 5 in, 1 out]
              }
              frame True {
                w254 = "Sim"
              }
            }
            "Mfg" <- w242
            "Model" <- w243
            "SN" <- w244
            "FW" <- w245
            n114 = call "Error.Set-Change Error Info.vi"("Std Code"=w239, "error in"=w236, "Description"="Failed or Lost Connection to Power Supply..") -> ("error out"=w237:errorcluster)  [unwired: 8 in]
          }
          frame "PS - Init" {
            w257 = T11 -5303 items=["No Error"=0, "Abort"=-2, "Misc"=-5000, "Fixture Error"=-5100, "File IO - General"=-5200, "FIle IO - Config Error"=-5201, "Instrument - General"=-5300, "Instrument - Serial Com"=-5301, "Instrument - Camera"=-5302, "Instrument - PS"=-5303, "Instrument - Oscilloscope"=-5304, "Instrument - Function Gen"=-5305, "Instrument - Load"=-5306, "Instrument - Meter"=-5307, "Instrument - Power Control"=-5308, "Instrument - Motion"=-5309, "Instrument - RF"=-5310, "System Exe"=-5400, "Image Processing"=-5500, "Communication"=-5600, "Script - Syntax Error"=-6000, "Script - Invalid Name or Param"=-6100, "Script - Timeout"=-6200, "Invalid Data"=-6300] ("Std Code")
            n115 = Unbundle By Name(w265) -> ("Cfg.Simulate"=w264:bool)
            n116 = Unbundle By Name(w260) -> ("Alias"=w267:refnum<visa-resource-name>, "Connected"=w263:bool)
            n117 = case shown="False" w264 {
              tunnel: w267 -> [w269 _]
              tunnel: [w271 _] -> w255
              tunnel: w263 -> [w270 _]
              frame False {
                n118 = case shown="True" w270 {
                  tunnel: w269 -> [w272 w274]
                  tunnel: [w272 w274] -> w268
                  tunnel: [_ w273] -> _
                  frame False {
                  }
                  frame True {
                    n119 = VISA Close(VISA resource name=w274) -> (error out=w273:errorcluster)  [unwired: 1 in]
                  }
                }
                n120 = VISA Open(VISA resource name=w268) -> (error out=w271:errorcluster)  [unwired: 4 in, 1 out]
              }
              frame True {
              }
            }
            n121 = Unbundle By Name(w255) -> ("status"=w262:bool)
            n122 = case shown="No Error" w255 {
              tunnel: w266 -> [w279 _]
              frame No Error {
                n123 = call <vilib>:"Q.Enqueue Task.vi"("Task Name"="PS - Get ID" ("Name"), "Q In"=w279) -> ("Q Out"=w278:refnum<queue>)  [unwired: 8 in, 1 out]
                n124 = To Variant(anything=FALSE) -> (Variant=w275:variant)
                n125 = call <vilib>:"Q.Enqueue Task.vi"("Data1"=w275, "Task Name"="PS - Set Output" ("Name"), "Q In"=w278) -> ()  [unwired: 7 in, 2 out]
              }
              frame Error {
              }
            }
            n126 = Not(x=w262) -> (.not. x?=w261:bool)
            n127 = Bundle By Name(cluster=w260, "Connected"=w261) -> (w259:T10)
            n128 = call "Error.Set-Change Error Info.vi"("Std Code"=w257, "error in"=w255, "Description"="Failed to Connect to Power Supply.") -> ("error out"=w256:errorcluster)  [unwired: 8 in]
          }
          frame "PS - Set Output" {
            w281 = T11 -5303 items=["No Error"=0, "Abort"=-2, "Misc"=-5000, "Fixture Error"=-5100, "File IO - General"=-5200, "FIle IO - Config Error"=-5201, "Instrument - General"=-5300, "Instrument - Serial Com"=-5301, "Instrument - Camera"=-5302, "Instrument - PS"=-5303, "Instrument - Oscilloscope"=-5304, "Instrument - Function Gen"=-5305, "Instrument - Load"=-5306, "Instrument - Meter"=-5307, "Instrument - Power Control"=-5308, "Instrument - Motion"=-5309, "Instrument - RF"=-5310, "System Exe"=-5400, "Image Processing"=-5500, "Communication"=-5600, "Script - Syntax Error"=-6000, "Script - Invalid Name or Param"=-6100, "Script - Timeout"=-6200, "Invalid Data"=-6300] ("Std Code")
            n129 = Variant To Data(type=FALSE, Variant=w289) -> (data=w286:bool, error out=w287:errorcluster)  [unwired: 1 in]
            n130 = case shown="No Error" w287 {
              tunnel: w286 -> [w294 _]
              tunnel: [w294 _] -> w285
              frame No Error {
              }
              frame Error {
              }
            }
            n131 = Unbundle By Name(w291) -> ("Cfg.Simulate"=w290:bool)
            n132 = Unbundle By Name(w293) -> ("Alias"=w292:refnum<visa-resource-name>)
            n133 = case shown="False" w290 {
              tunnel: w292 -> [w299 _]
              tunnel: [w300 _] -> w283
              tunnel: w285 -> [w298 _]
              frame False {
                n134 = call "DSPS_E36000.Set Output Voltage.vi"("CurLim"="Current Lim", "State"=w298, "Voltage"="Voltage", "VISA Alias"=w299) -> ("error out"=w300:errorcluster)  [unwired: 6 in, 1 out]
              }
              frame True {
              }
            }
            n135 = case shown="No Error" w283 {
              tunnel: w285 -> [w295 _]
              frame No Error {
                "PS Output State" <- w295
              }
              frame Error {
              }
            }
            n136 = call "Error.Set-Change Error Info.vi"("Std Code"=w281, "error in"=w283, "Description"="Failed or Lost Connection to Power Supply.") -> ("error out"=w284:errorcluster)  [unwired: 8 in]
          }
          frame "Return" {
            n137 = Variant To Data(type="", Variant=w302) -> (data=w307:string, error out=w306:errorcluster)  [unwired: 1 in]
            n138 = case shown="No Error" w306 {
              selector: w306 -> [_ w319]
              tunnel: w307 -> [w316 _]
              tunnel: [w314 w319] -> w303
              tunnel: w305 -> [w313 w318]
              tunnel: [w312 w318] -> w304
              tunnel: w301 -> [w310 _]
              frame No Error {
                n139 = Unbundle By Name(w313) -> ("FunctMgr"=w317:refnum<class "FunctMgr.lvclass">, "Local Error"=w311:errorcluster)
                n140 = call "FunctMgr.Pop and Return.vi"("error in (no error)"=w311, "Data"=w310, "Ret ID"=w316, "FunctMgr in"=w317) -> ("error out"=w314:errorcluster, "FunctMgr out"=w315:refnum<class "FunctMgr.lvclass">)  [unwired: 5 in, 1 out]
                n141 = Bundle By Name(cluster=w313, "FunctMgr"=w315) -> (w312:T10)
              }
              frame Error {
                # "Can't Return.  Invalid ID."
              }
            }
          }
          frame "Save Current to File" {
            w334 = T12 2 items=["User Home"=0, "User Desktop"=1, "User Documents"=2, "User Application Data"=3, "User Preferences"=4, "User Temporary"=5, "Public Documents"=6, "Public Application Data"=7, "Public Preferences"=8, "Public Cache"=13, "System Core Libraries"=9, "System Installed Libraries"=10, "Application Files"=11, "Boot Volume Root"=12] ("system directory type")
            n142 = Unbundle By Name(w344) -> ("GraphData.t"=w321:dbl[], "GraphData.Y"=w330:dbl[])
            n143 = Number To Fractional String(number=w330) -> (F-format string=w329:string[])  [unwired: 3 in]
            n144 = Number To Fractional String(number=w321) -> (F-format string=w320:string[])  [unwired: 3 in]
            n145 = Format Date/Time String(time format string (%c)="PS Current Data, %H%M%S_%m%d%Y.csv" ("prompt (Choose or enter file path)")) -> (date/time string=w332:string)  [unwired: 2 in]
            n146 = call <vilib>:"Get System Directory.vi"("system directory type"=w334) -> ("system directory"=w333:path)  [unwired: 10 in]
            n147 = Build Path(base path=w333, name or relative path=w332) -> (appended path=w331:path)
            n148 = Open/Create/Replace File(file path (use dialog)=w331, operation (0:open)=T7."replace or create") -> (refnum out=w340:refnum<file>, cancelled=w336:bool, error out=w343:errorcluster)  [unwired: 4 in]
            n149 = Build Array(w320, w329) -> (w328:string[][])
            n150 = Transpose 2D Array(2D array=w328) -> (transposed array=w326:string[][])
            n151 = Build Array (concatenate)(string[] ["Time", "Current(A)"], w326) -> (w325:string[][])
            n152 = Array To Spreadsheet String(delimiter (Tab)=",", array=w325, 3:"" ("format string")) -> (spreadsheet string=w322:string)
            n153 = Write to Text File(file (use dialog)=w340, text=w322, error in=w343) -> (refnum out=w341:refnum<file>, error out=w342:errorcluster)  [unwired: 1 in, 1 out]
            n154 = Close File(refnum=w341, error in=w342) -> (path=w339:path, error out=w338:errorcluster)
            n155 = case shown="False" w336 {
              tunnel: w339 -> [w347 _]
              tunnel: w338 -> [w346 _]
              frame False {
                n156 = call <vilib>:"File.Open File or Folder.vi"("Error In"=w346, "Path"=w347) -> ()  [unwired: 9 in, 1 out]
              }
              frame True {
              }
            }
          }
          frame "Set Alias" {
            n157 = local read "Alias"() -> (w348:refnum<visa-resource-name>)
            n158 = Bundle By Name(cluster=w350, "Alias"=w348) -> (w349:T10)
          }
          frame "Simulate" {
            # "Reset to restart in new simulate state"
            # "Forward Simulate state to child modules"
            n159 = Variant To Data(type=FALSE, Variant=w363) -> (data=w353:bool)  [unwired: 1 in, 1 out]
            n160 = Unbundle By Name(w356) -> ("Cfg.Is Child?"=w352:bool, "Cfg.Dirs.Config"=w355:path, "SW Rev.AppName"=w354:string)
            n161 = call <vilib>:"Q.Enqueue Reset.vi"("Q In"=w357) -> ()  [unwired: 9 in, 2 out]
            n162 = case shown="False" w352 {
              tunnel: w355 -> [w365 _]
              tunnel: w354 -> [_ _]
              tunnel: w353 -> [w364 _]
              frame False {
                n163 = call <vilib>:"Config.Simulate.Set.vi"("Simulate"=w364, "Config Folder"=w365) -> ()  [unwired: 9 in, 1 out]
              }
              frame True {
              }
            }
            n164 = Bundle By Name(cluster=w356, "Cfg.Simulate"=w353) -> (w361:T5)
            n165 = property on="Simulate Indication" class="Str"("Visible"=w353) -> ()  [unwired: 2 in, 2 out]
            n166 = Unbundle By Name(w360) -> ("App.Child Modules"=w359:cluster{"VI Ref":refnum<vi>, "Name":string}[])
            n167 = To Variant(anything=w353) -> (Variant=w358:variant)
            n168 = for {
              tunnel: w359 -> [w369] mode=indexing
              tunnel: w358 -> [w366]
              n169 = Unbundle By Name(w369) -> ("Name"=w368:string)
              n170 = call <vilib>:"Q.Enqueue Task.vi"("Data1"=w366, "Q Name"=w368, "Task Name"="Simulate") -> ()  [unwired: 7 in, 2 out]
            }
          }
          frame "Simulate - Toggle" {
            n171 = call <vilib>:"Q.Enqueue Reset.vi"("Q In"=w375) -> ()  [unwired: 9 in, 2 out]
            n172 = Unbundle By Name(w372) -> ("Cfg.Simulate"=w371:bool)
            n173 = Not(x=w371) -> (.not. x?=w370:bool)
            n174 = Bundle By Name(cluster=w372, "Cfg.Simulate"=w370) -> (w373:T5)
            n175 = property on="Simulate Indication" class="Str"("Visible"=w370) -> ()  [unwired: 2 in, 2 out]
          }
          frame "Status" {
            n176 = Variant To Data(type="", Variant=w379) -> (data=w381:string, error out=w380:errorcluster)  [unwired: 1 in]
            n177 = case shown="No Error" w380 {
              selector: w380 -> [_ w387]
              tunnel: w378 -> [w386 _]
              tunnel: w377 -> [_ _]
              tunnel: w381 -> [w384 _]
              tunnel: [_ w387] -> w376
              frame No Error {
                # "Received from Child\nOnly write to status indicator (not event log)\nChild already recorded to event log."
                n178 = Unbundle By Name(w386) -> ("Log"=w385:refnum<class "Event Notification.lvclass">)
                n179 = call <vilib>:"Event Notification.Status Message.vi"("Log"=FALSE, "Message"=w384, "Event Notification in"=w385) -> ()  [unwired: 9 in]
              }
              frame Error {
              }
            }
          }
          frame Default {
            n180 = call <vilib>:"Module.Default Tasks.vi"("Sys"=w389, "error in"=w391, "Data2"=w392, "Data1"=w393, "Sub"=w394) -> ("error out"=w390:errorcluster, "Sys Out"=w388:T5)  [unwired: 5 in]
          }
        }
      }
      frame "Function" {
        # "Return by default"
        n181 = case shown="Default" w404 {
          selector: w404 -> [_ _ _ _ _ _ _ w578]
          tunnel: w408 -> [w422 w437 w473 w480 w491 w529 w552 w582]
          tunnel: w407 -> [w421 w436 w472 w479 w493 w536 w567 w583]
          tunnel: [w422 w437 w473 w480 w491 w529 w552 w582] -> w406
          tunnel: [w421 w436 w472 w479 w493 w536 w567 w583] -> w405
          tunnel: w403 -> [w419 _ _ w478 w497 _ w551 _]
          tunnel: w402 -> [w420 _ _ _ _ _ w554 w579]
          tunnel: w401 -> [_ _ _ _ _ _ _ _]
          tunnel: w399 -> [_ _ _ _ _ _ _ w577]
          tunnel: [w415 w429 w463 w474 w492 w525 _ w576] -> w398
          tunnel: [_ w440 w464 _ _ w533 _ variant] -> w397
          tunnel: [FALSE _ _ _ _ _ _ FALSE] -> w396
          frame "Lock Controls" {
            n182 = Variant To Data(type=FALSE, Variant=w419) -> (data=w417:bool, error out=w416:errorcluster)  [unwired: 1 in]
            n183 = case shown="No Error" w416 {
              selector: w416 -> [_ w427]
              tunnel: w420 -> [w424 _]
              tunnel: w417 -> [w423 _]
              tunnel: [_ w427] -> w415
              frame No Error {
                n184 = To Variant(anything=w423) -> (Variant=w426:variant)
                n185 = call <vilib>:"Q.Enqueue Task.vi"("Data1"=w426, "Task Name"="Lock Test Controls", "Q In"=w424) -> ()  [unwired: 7 in, 2 out]
              }
              frame Error {
              }
            }
          }
          frame "PS_GetID" {
            w431 = T11 -5303 items=["No Error"=0, "Abort"=-2, "Misc"=-5000, "Fixture Error"=-5100, "File IO - General"=-5200, "FIle IO - Config Error"=-5201, "Instrument - General"=-5300, "Instrument - Serial Com"=-5301, "Instrument - Camera"=-5302, "Instrument - PS"=-5303, "Instrument - Oscilloscope"=-5304, "Instrument - Function Gen"=-5305, "Instrument - Load"=-5306, "Instrument - Meter"=-5307, "Instrument - Power Control"=-5308, "Instrument - Motion"=-5309, "Instrument - RF"=-5310, "System Exe"=-5400, "Image Processing"=-5500, "Communication"=-5600, "Script - Syntax Error"=-6000, "Script - Invalid Name or Param"=-6100, "Script - Timeout"=-6200, "Invalid Data"=-6300] ("Std Code")
            n186 = Unbundle By Name(w437) -> ("Cfg.Simulate"=w438:bool)
            n187 = Unbundle By Name(w436) -> ("Alias"=w439:refnum<visa-resource-name>)
            n188 = case shown="False" w438 {
              tunnel: w439 -> [w450 _]
              tunnel: [w455 _] -> w428
              tunnel: [w454 w456] -> w432
              tunnel: [w453 w456] -> w433
              tunnel: [w452 w456] -> w434
              tunnel: [w451 w456] -> w435
              frame False {
                n189 = call "DSPS_E36000.Get ID.vi"("VISA Alias"=w450) -> ("error out"=w455:errorcluster, "SN"=w453:string, "Model"=w452:string, "FW"=w454:string, "Mfg"=w451:string)  [unwired: 5 in, 1 out]
              }
              frame True {
                w456 = "Sim"
              }
            }
            n190 = local write "Model"(w434) -> ()
            n191 = local write "SN"(w433) -> ()
            n192 = local write "Mfg"(w435) -> ()
            n193 = Build Array("PS_Model", w434) -> (w447:string[])
            n194 = Build Array("PS_SN", w433) -> (w448:string[])
            n195 = Build Array("PS_FW", w432) -> (w449:string[])
            n196 = Build Array("PS_Mfg", w435) -> (w446:string[])
            n197 = local write "FW"(w432) -> ()
            n198 = call "Error.Set-Change Error Info.vi"("Std Code"=w431, "error in"=w428, "Description"="Failed or Lost Connection to Power Supply.") -> ("error out"=w429:errorcluster)  [unwired: 8 in]
            n199 = Build Array(w446, w447, w448, w449) -> (w441:string[][])
            n200 = To Variant(anything=w441) -> (Variant=w440:variant)
            n201 = local write "Error"(w429) -> ()
          }
          frame "GetCurrentMetrics" {
            n202 = local read "CurrPeak(A)"() -> (w460:dbl)
            n203 = local read "Current(A)"() -> (w462:dbl)
            n204 = local read "CurrAvg(A)"() -> (w461:dbl)
            n205 = Number To Fractional String(number=w461) -> (F-format string=w458:string)  [unwired: 3 in]
            n206 = Number To Fractional String(number=w462) -> (F-format string=w459:string)  [unwired: 3 in]
            n207 = Number To Fractional String(number=w460) -> (F-format string=w457:string)  [unwired: 3 in]
            n208 = Build Array("AverageCurrent_A", w458) -> (w470:string[])
            n209 = Build Array("Current_A", w459) -> (w469:string[])
            n210 = Build Array("PeakCurrent_A", w457) -> (w471:string[])
            n211 = Build Array(w469, w470, w471) -> (w465:string[][])
            n212 = To Variant(anything=w465) -> (Variant=w464:variant)
            n213 = local read "Error"() -> (w463:errorcluster)
          }
          frame "PS_SetCurrentAvgCnt" {
            n214 = Variant To Data(type=string[] [], Variant=w478) -> (data=w475:string[], error out=w476:errorcluster)  [unwired: 1 in]
            n215 = case shown="Error" w476 {
              tunnel: w475 -> [w486 _]
              tunnel: [_ w488] -> w474
              frame No Error {
                n216 = Index Array(array=w486) -> (element=w485:string)  [unwired: 1 in]
                n217 = Decimal String To Number(string=w485) -> (number=w484:i32)  [unwired: 2 in, 1 out]
                n218 = In Range and Coerce(upper limit=1000, x=w484, lower limit=1) -> (coerced(x)=w481:i32)  [unwired: 1 out]
                n219 = local write "Average Cnt"(w481) -> ()
              }
              frame Error {
                w489 = T11 -6000 items=["No Error"=0, "Abort"=-2, "Misc"=-5000, "Fixture Error"=-5100, "File IO - General"=-5200, "FIle IO - Config Error"=-5201, "Instrument - General"=-5300, "Instrument - Serial Com"=-5301, "Instrument - Camera"=-5302, "Instrument - PS"=-5303, "Instrument - Oscilloscope"=-5304, "Instrument - Function Gen"=-5305, "Instrument - Load"=-5306, "Instrument - Meter"=-5307, "Instrument - Power Control"=-5308, "Instrument - Motion"=-5309, "Instrument - RF"=-5310, "System Exe"=-5400, "Image Processing"=-5500, "Communication"=-5600, "Script - Syntax Error"=-6000, "Script - Invalid Name or Param"=-6100, "Script - Timeout"=-6200, "Invalid Data"=-6300] ("Std Code")
                n220 = call "Error.Set-Change Error Info.vi"("Std Code"=w489, "Description"="Invalid Function Data Type, Expected 1D Array of String.", "Set Error"=TRUE) -> ("error out"=w488:errorcluster)  [unwired: 8 in]
              }
            }
          }
          frame "PS_SetOutput" {
            n221 = Variant To Data(type=string[] [], Variant=w497) -> (data=w494:string[], error out=w495:errorcluster)  [unwired: 1 in]
            n222 = case shown="No Error" w495 {
              tunnel: w494 -> [w509 _]
              tunnel: w493 -> [w508 _]
              tunnel: [w499 w520] -> w492
              tunnel: w491 -> [w504 _]
              frame No Error {
                w500 = T11 -5303 items=["No Error"=0, "Abort"=-2, "Misc"=-5000, "Fixture Error"=-5100, "File IO - General"=-5200, "FIle IO - Config Error"=-5201, "Instrument - General"=-5300, "Instrument - Serial Com"=-5301, "Instrument - Camera"=-5302, "Instrument - PS"=-5303, "Instrument - Oscilloscope"=-5304, "Instrument - Function Gen"=-5305, "Instrument - Load"=-5306, "Instrument - Meter"=-5307, "Instrument - Power Control"=-5308, "Instrument - Motion"=-5309, "Instrument - RF"=-5310, "System Exe"=-5400, "Image Processing"=-5500, "Communication"=-5600, "Script - Syntax Error"=-6000, "Script - Invalid Name or Param"=-6100, "Script - Timeout"=-6200, "Invalid Data"=-6300] ("Std Code")
                # "If error, add description."
                n223 = Unbundle By Name(w504) -> ("Cfg.Simulate"=w503:bool)
                n224 = Unbundle By Name(w508) -> ("Alias"=w505:refnum<visa-resource-name>)
                n225 = Index Array(array=w509) -> (element #1=w512:string, element #2=w511:string, element #3=w510:string)  [unwired: 3 in]
                n226 = call <vilib>:"Trim Whitespace.vi"("string"=w512) -> ("trimmed string"=w514:string)  [unwired: 1 in]
                n227 = Equal?(x="1", y=w514) -> (x = y?=w502:bool)
                n228 = Fract/Exp String To Number(string=w511) -> (number=w506:dbl)  [unwired: 3 in, 1 out]
                n229 = Fract/Exp String To Number(string=w510) -> (number=w507:dbl)  [unwired: 3 in, 1 out]
                n230 = case shown="False" w503 {
                  tunnel: w502 -> [w515 _]
                  tunnel: w507 -> [w519 _]
                  tunnel: w506 -> [w518 _]
                  tunnel: w505 -> [w517 _]
                  tunnel: [w516 _] -> w498
                  frame False {
                    n231 = call "DSPS_E36000.Set Output Voltage.vi"("CurLim"=w519, "State"=w515, "Voltage"=w518, "VISA Alias"=w517) -> ("error out"=w516:errorcluster)  [unwired: 6 in, 1 out]
                  }
                  frame True {
                  }
                }
                n232 = local write "Current Lim"(w507) -> ()
                n233 = local write "Voltage"(w506) -> ()
                n234 = local write "PS Output State"(w502) -> ()
                n235 = call "Error.Set-Change Error Info.vi"("Std Code"=w500, "error in"=w498, "Description"="Failed or Lost Connection to Power Supply.") -> ("error out"=w499:errorcluster)  [unwired: 8 in]
              }
              frame Error {
                w522 = T11 -6000 items=["No Error"=0, "Abort"=-2, "Misc"=-5000, "Fixture Error"=-5100, "File IO - General"=-5200, "FIle IO - Config Error"=-5201, "Instrument - General"=-5300, "Instrument - Serial Com"=-5301, "Instrument - Camera"=-5302, "Instrument - PS"=-5303, "Instrument - Oscilloscope"=-5304, "Instrument - Function Gen"=-5305, "Instrument - Load"=-5306, "Instrument - Meter"=-5307, "Instrument - Power Control"=-5308, "Instrument - Motion"=-5309, "Instrument - RF"=-5310, "System Exe"=-5400, "Image Processing"=-5500, "Communication"=-5600, "Script - Syntax Error"=-6000, "Script - Invalid Name or Param"=-6100, "Script - Timeout"=-6200, "Invalid Data"=-6300] ("Std Code")
                n236 = call "Error.Set-Change Error Info.vi"("Std Code"=w522, "Description"="Invalid Function Data Type, Expected 1D Array of String.", "Set Error"=TRUE) -> ("error out"=w520:errorcluster)  [unwired: 8 in]
              }
            }
          }
          frame "PS_GetCurrent" {
            w527 = T11 -5303 items=["No Error"=0, "Abort"=-2, "Misc"=-5000, "Fixture Error"=-5100, "File IO - General"=-5200, "FIle IO - Config Error"=-5201, "Instrument - General"=-5300, "Instrument - Serial Com"=-5301, "Instrument - Camera"=-5302, "Instrument - PS"=-5303, "Instrument - Oscilloscope"=-5304, "Instrument - Function Gen"=-5305, "Instrument - Load"=-5306, "Instrument - Meter"=-5307, "Instrument - Power Control"=-5308, "Instrument - Motion"=-5309, "Instrument - RF"=-5310, "System Exe"=-5400, "Image Processing"=-5500, "Communication"=-5600, "Script - Syntax Error"=-6000, "Script - Invalid Name or Param"=-6100, "Script - Timeout"=-6200, "Invalid Data"=-6300] ("Std Code")
            # "If error, add description."
            n237 = local read "Continuous Read"() -> (w528:bool)
            n238 = case shown="True" w528 {
              tunnel: w536 -> [w542 w550]
              tunnel: [w541 _] -> w524
              tunnel: [w539 w549] -> w530
              tunnel: w529 -> [w538 _]
              frame False {
                n239 = Unbundle By Name(w538) -> ("Cfg.Simulate"=w537:bool)
                n240 = Unbundle By Name(w542) -> ("Alias"=w540:refnum<visa-resource-name>)
                n241 = case shown="False" w537 {
                  tunnel: [w545 _] -> w541
                  tunnel: w540 -> [w544 _]
                  tunnel: [w543 w546] -> w539
                  frame False {
                    n242 = call "DSPS_E36000.Get Current.vi"("VISA Alias"=w544) -> ("error out"=w545:errorcluster, "Current"=w543:dbl)  [unwired: 7 in, 2 out]
                  }
                  frame True {
                    n243 = Random Number (0-1)() -> (number: 0 to 1=w548:dbl)
                    n244 = Multiply(x=w548, y=0.8) -> (x*y=w546:dbl)
                  }
                }
                n245 = local write "Current(A)"(w539) -> ()
              }
              frame True {
                n246 = Unbundle By Name(w550) -> ("Current"=w549:dbl)
              }
            }
            n247 = Number To Fractional String(number=w530) -> (F-format string=w535:string)  [unwired: 3 in]
            n248 = Build Array("Current_A", w535) -> (w532:string[])
            n249 = call "Error.Set-Change Error Info.vi"("Std Code"=w527, "error in"=w524, "Description"="Failed or Lost Connection to Power Supply.") -> ("error out"=w525:errorcluster)  [unwired: 8 in]
            n250 = Build Array(w532) -> (w531:string[][])
            n251 = To Variant(anything=w531) -> (Variant=w533:variant)
          }
          frame "CurrentMonitor" {
            n252 = Variant To Data(type=string[] [] ("appended array"), Variant=w551) -> (data=w564:string[], error out=w565:errorcluster)  [unwired: 1 in]
            n253 = case shown="No Error" w565 {
              tunnel: w564 -> [w575 _]
              tunnel: [w574 _] -> w563
              frame No Error {
                n254 = Index Array(array=w575) -> (element=w574:string)  [unwired: 1 in]
              }
              frame Error {
              }
            }
            n255 = call <vilib>:"Trim Whitespace.vi"("string"=w563) -> ("trimmed string"=w561:string)  [unwired: 1 in]
            n256 = Equal?(x="1", y=w561) -> (x = y?=w558:bool)
            n257 = case shown="True" w558 {
              tunnel: [FALSE ("Current Read") TRUE ("Current Read")] -> w553
              tunnel: w554 -> [_ w570]
              frame False {
              }
              frame True {
                n258 = call <vilib>:"Q.Enqueue Task.vi"("Task Name"="Current Graph - Clear", "Q In"=w570) -> ("Q Out"=w571:refnum<queue>)  [unwired: 8 in, 1 out]
                n259 = call <vilib>:"Q.Enqueue Task.vi"("Task Name"="PS - Get Current", "Q In"=w571) -> ()  [unwired: 8 in, 2 out]
              }
            }
            n260 = Select(t="Monitoring Input Current", s=w558, f="Stopped Current Monitoring") -> (s? t:f=w557:string)
            n261 = Unbundle By Name(w552) -> ("Log"=w560:refnum<class "Event Notification.lvclass">)
            n262 = call <vilib>:"Event Notification.Status Message.vi"("Log"=FALSE, "Message"=w557, "Event Notification in"=w560) -> ()  [unwired: 9 in]
            n263 = local write "Continuous Read"(w553) -> ()
          }
          frame Default {
            n264 = call <vilib>:"SeqMgr.Error, Build Function Name Error Message.vi"("Data2"=w577, "Funct_Seq Name"=w578, "Local Q"=w579) -> ("error out"=w576:errorcluster)  [unwired: 8 in]
          }
        }
        n265 = case shown="False" w396 {
          tunnel: [w412 w413] -> w400
          tunnel: w399 -> [w411 _]
          tunnel: w398 -> [w410 w413]
          tunnel: w397 -> [w409 _]
          frame False {
            n266 = call <vilib>:"Q.Return Function Data.vi"("error in"=w410, "Data2"=w411, "Ret Data"=w409) -> ("error out"=w412:errorcluster)  [unwired: 8 in]
          }
          frame True {
          }
        }
      }
      frame "App" {
        n267 = case shown="\"Set Logging Level\"" w591 {
          tunnel: w590 -> [_ _]
          tunnel: w589 -> [_ w603]
          tunnel: w588 -> [_ _]
          tunnel: w587 -> [w593 w600]
          tunnel: w586 -> [w592 w602]
          tunnel: [w593 w601] -> w585
          tunnel: [w592 w602] -> w584
          frame Default {
          }
          frame "Set Logging Level" {
            n268 = Variant To Data(type=Event_Log.Log_Level."Normal" ("Log Level"), Variant=w603) -> (data=w596:T1)  [unwired: 1 in, 1 out]
            n269 = local read "Logging Level"() -> (w595:T1)
            n270 = Unbundle By Name(w600) -> ("Log"=w598:refnum<class "Event Notification.lvclass">)
            n271 = Not Equal?(x=w596, y=w595) -> (x != y?=w594:bool)
            n272 = call <vilib>:"Event Notification.Set Logging Level.vi"("Log Level"=w596, "Event Notification in"=w598) -> ("Event Notification out"=w599:refnum<class "Event Notification.lvclass">)  [unwired: 9 in]
            n273 = case shown="True" w594 {
              tunnel: w596 -> [_ w604]
              frame False {
              }
              frame True {
                n274 = local write "Logging Level"(w604) -> ()
              }
            }
            n275 = Bundle By Name(cluster=w600, "Log"=w599) -> (w601:T5)
          }
        }
      }
      frame "Error", Default {
        n276 = case shown="\"Error\"" w612 {
          selector: w612 -> [_ w664]
          tunnel: [_ w665] -> w613
          tunnel: w611 -> [w622 _]
          tunnel: w610 -> [w620 _]
          tunnel: w609 -> [w621 _]
          tunnel: w608 -> [w619 _]
          tunnel: w606 -> [w616 w663]
          tunnel: w607 -> [w617 _]
          tunnel: [w615 w663] -> w605
          frame "Error" {
            n277 = case shown="\"Clear\"" w621 {
              tunnel: w622 -> [_ w661 _]
              tunnel: w620 -> [w657 _ _]
              tunnel: [w657 w659 _] -> w614
              tunnel: w619 -> [w656 w658 w662]
              tunnel: [w656 w658 w662] -> w618
              frame Default {
              }
              frame "Error" {
                n278 = Variant To Data(type=errorcluster {"status"=FALSE, "code"=0, "source"=""} ("error constant"), Variant=w661) -> (data=w659:errorcluster)  [unwired: 1 in, 1 out]
              }
              frame "Clear" {
              }
            }
            n279 = case shown="Error" w614 {
              selector: w614 -> [_ w635]
              tunnel: w618 -> [_ _]
              tunnel: w617 -> [w625 w638]
              tunnel: w616 -> [w628 w647]
              tunnel: [w627 w646] -> w615
              frame No Error {
                # "Clear Local Errors"
                n280 = Unbundle By Name(w628) -> ("Local Error"=w630:errorcluster)
                n281 = Unbundle By Name(w625) -> ("Log"=w624:refnum<class "Event Notification.lvclass">)
                n282 = case shown="Error" w630 {
                  tunnel: w624 -> [_ w634]
                  frame No Error {
                  }
                  frame Error {
                    n283 = call <vilib>:"Event Notification.Status Message.vi"("Display"=TRUE, "Level"=Event_Log.Log_Level."Normal", "Message"="Cleared Errors", "Event Notification in"=w634) -> ()  [unwired: 8 in]
                  }
                }
                n284 = control-ref of="Error Status"() -> (w626:refnum<vi>)
                n285 = invoke on="Error" class="Clust (strict)" method="Reinit To Default"() -> ()  [unwired: 3 in, 3 out]
                n286 = property on="Clear Error" class="Bool"("Visible"=FALSE) -> ()  [unwired: 2 in, 2 out]
                n287 = call <vilib>:"Status.Simple Text Status Indicator.vi"("Status TextBox"=w626) -> ()  [unwired: 10 in, 1 out]
                n288 = Bundle By Name(cluster=w628, "Local Error"=errorcluster {"status"=FALSE, "code"=0, "source"=""}) -> (w627:T10)
              }
              frame Error {
                # "Record Error"
                n289 = Unbundle By Name(w647) -> ("Local Error"=w645:errorcluster)
                n290 = Unbundle By Name(w638) -> ("Log"=w642:refnum<class "Event Notification.lvclass">)
                n291 = Unbundle By Name(w635) -> ("code"=w649:i32, "source"=w648:string)
                n292 = Unbundle By Name(w638) -> ("Cfg.Is Child?"=w637:bool, "Cfg.Parent Q"=w636:refnum<queue>)
                n293 = Format Into String(format string="ERROR!!! Code: %d, Desc: %s", w649, w648) -> (resulting string=w641:string)  [unwired: 2 in, 1 out]
                n294 = control-ref of="Error Status"() -> (w643:refnum<vi>)
                n295 = property on="Clear Error" class="Bool"("Visible"=TRUE) -> ()  [unwired: 2 in, 2 out]
                n296 = Merge Errors(w645, w635) -> (w644:errorcluster)
                n297 = call <vilib>:"Event Notification.Status Message with Error In.vi"("Type"=Event_Log.Notification_Type."Error", "Message"=w641, "Event Notification in"=w642) -> ()  [unwired: 9 in]
                n298 = call <vilib>:"Status.Simple Text Status Indicator.vi"("error in"=w635, "Status TextBox"=w643) -> ()  [unwired: 9 in, 1 out]
                n299 = case shown="True" w637 {
                  tunnel: w636 -> [_ w655]
                  tunnel: w635 -> [_ w654]
                  tunnel: [_ w651] -> _
                  frame False {
                  }
                  frame True {
                    w652 = "Error"
                    n300 = To Variant(anything=w654) -> (Variant=w653:variant)
                    n301 = call <vilib>:"Q.Enqueue Item.vi"("Data1"=w653, "Sub"=w652, "Cmd"=w652, "Q In"=w655) -> ("error out"=w651:errorcluster)  [unwired: 6 in, 1 out]
                  }
                }
                n302 = Bundle By Name(cluster=w647, "Local Error"=w644) -> (w646:T10)
                "Error" <- w635
              }
            }
          }
          frame Default {
            n303 = Concatenate Strings("Undefined State: \"", w664, "\".") -> (w666:string)
            n304 = Bundle By Name(cluster=errorcluster {"status"=TRUE, "code"=-5000, "source"=""} ("error constant"), "source"=w666) -> (w665:errorcluster)
          }
        }
      }
      frame "Exit" {
        # "This connection is made to not close\n the module until exit tasks are done."
        n305 = stacked-sequence {
          tunnel: w671 -> [w680 w682]
          tunnel: [errorcluster {"status"=FALSE, "code"=0, "source"=""} ("error constant") _] -> w670
          frame #0 {
            # "Close connection to instruments"
            n306 = Unbundle By Name(w680) -> ("Alias"=w678:refnum<visa-resource-name>)
            n307 = call "DSPS_E36000.Set Output Voltage.vi"("State"=FALSE, "VISA Alias"=w678) -> ("error out"=w676:errorcluster, "VISA Alias Dup"=w675:refnum<visa-resource-name>)  [unwired: 8 in]
            n308 = VISA Close(VISA resource name=w675, error in (no error)=w676) -> (error out=w679:errorcluster)
            n309 = call <vilib>:"Clear Errors.vi"("error in (no error)"=w679) -> ()  [unwired: 5 in, 2 out]
          }
          frame #1 {
            # "Leave error not connected\nIgnore errors"
            # "Send Exit command to child modules"
            n310 = Unbundle By Name(w682) -> ("App.Child Modules"=w683:cluster{"VI Ref":refnum<vi>, "Name":string}[])
            n311 = for {
              tunnel: w683 -> [w686] mode=indexing
              tunnel: [w684] -> _ mode=indexing
              n312 = Unbundle By Name(w686) -> ("Name"=w685:string)
              n313 = call <vilib>:"Q.Enqueue Exit.vi"("Q Name"=w685) -> ("error out"=w684:errorcluster)  [unwired: 9 in, 1 out]
            }
          }
        }
        n314 = call <vilib>:"Module.Destructor.vi"("error in"=w670, "Sys"=w672) -> ("error out"=w674:errorcluster)  [unwired: 9 in]
      }
    }
  }
  n315 = while "Event Loop" {
    tunnel: w7 -> [w689]
    stop <- w690 stop-if-true
    n316 = Unbundle By Name(w689) -> ("Stop.Ref"=w688:refnum<event-registration>, "Main Q"=w687:refnum<queue>)
    n317 = event shown="[14] \"Continuous Read\": Value Change" {
      selector: w688 -> [_ _ _ _ _ _ _ _ _ _ _ _ _ _ _]
      dyn-events: _ -> [_ _ _ _ _ _ _ _ _ _ _ _ _ _ _]
      timeout: _ -> [_ _ _ _ _ _ _ _ _ _ _ _ _ _ _]
      tunnel: [w693 _ _ w711 TRUE _ _ _ _ _ _ _ _ _ _] -> w690
      tunnel: w689 -> [w692 _ _ w709 _ _ _ _ _ _ _ _ _ _ _]
      tunnel: w687 -> [w695 w705 _ w710 _ w733 w734 w736 w738 w741 w745 w747 w749 w754 w756]
      event Panel Close? {
        n318 = event-data() -> ()  [unwired: 1 in, 4 out]
        n319 = Unbundle By Name(w692) -> ("Cfg.Is Child?"=w691:bool)
        n320 = case shown="True" w691 {
          tunnel: w695 -> [w698 w701]
          tunnel: [TRUE TRUE] -> w694
          tunnel: [TRUE FALSE] -> w693
          tunnel: [_ w699] -> _
          frame False {
            # "Parent - Exit"
            n321 = call <vilib>:"Q.Enqueue Exit.vi"("Q In"=w698) -> ()  [unwired: 9 in, 2 out]
          }
          frame True {
            # "Child - Hide Panel and if was \nin a subpanel, return to subpanel."
            n322 = call <vilib>:"Module.Window, Q Task.vi"("Action"=Window.Task,_Action."Return to SubPanel()", "Q In"=w701) -> ("error out"=w699:errorcluster)  [unwired: 8 in, 1 out]
          }
        }
        n323 = event-data("Discard?"=w694) -> ()  [unwired: 1 in, 1 out]
      }
      event Panel Resize {
        n324 = event-data() -> ()  [unwired: 1 in, 8 out]
        n325 = call <vilib>:"Module.Window, Q Task.vi"("Action"=Window.Task,_Action."Resize()", "Q In"=w705) -> ()  [unwired: 8 in, 2 out]
      }
      event "Leave Maint": Value Change {
        n326 = event-data() -> ()  [unwired: 1 in, 6 out]
        n327 = local write "Main Tab"(0) -> ()
      }
      event Menu Selection (User) {
        n328 = event-data() -> ("MenuRef"=w707:refnum<k9>, "ItemTag"=w708:string)  [unwired: 1 in, 5 out]
        n329 = case shown="\"Help.About\"" w708 {
          selector: w708 -> [w713 _ _ _ _ w723 _ _]
          tunnel: [_ TRUE _ _ _ _ _ _] -> w711
          tunnel: w710 -> [_ w716 _ w719 _ w727 w729 w731]
          tunnel: [_ _ w718 _ _ _ _ _] -> _
          tunnel: w709 -> [w712 _ _ _ w721 _ _ _]
          tunnel: w707 -> [_ _ _ _ _ w724 _ _]
          frame Default {
            # "Check if a help document was selected.\nIf so, open the document"
            n330 = Unbundle By Name(w712) -> ("Docs.Tags"=w715:string[], "Docs.Paths"=w714:path[])
            n331 = call <vilib>:"Menu.Help, Open User Manual Items.vi"("Menu Tag Selection"=w713, "Paths"=w714, "Tags"=w715) -> ()  [unwired: 8 in, 1 out]
          }
          frame "Exit" {
            n332 = call <vilib>:"Q.Enqueue Exit.vi"("Q In"=w716) -> ()  [unwired: 9 in, 2 out]
          }
          frame "Event Log" {
            n333 = call <vilib>:"Event Log.Show.vi"() -> ("error out"=w718:errorcluster)  [unwired: 11 in]
          }
          frame "Reset" {
            n334 = call <vilib>:"Q.Enqueue Reset.vi"("Q In"=w719) -> ()  [unwired: 9 in, 2 out]
          }
          frame "Help.About" {
            n335 = Unbundle By Name(w721) -> ("SW Rev"=w720:T4)
            n336 = call <vilib>:"Help.About.vi"("SW Version"=w720) -> ()  [unwired: 11 in]
          }
          frame "Simulate OFF", "Simulate ON" {
            n337 = call <vilib>:"Menu.Simulate, Set Menu State.vi"("Menu Tag"=w723, "Menu Ref"=w724) -> ("Sim ON"=w722:bool)  [unwired: 8 in, 1 out]
            n338 = To Variant(anything=w722) -> (Variant=w726:variant)
            n339 = call <vilib>:"Q.Enqueue Task.vi"("Data1"=w726, "Task Name"="Simulate", "Q In"=w727) -> ()  [unwired: 7 in, 2 out]
          }
          frame "Show Block Diagram" {
            n340 = call <vilib>:"Module.Window, Q Task.vi"("Action"=Window.Task,_Action."Open Block Diagram()", "Q In"=w729) -> ()  [unwired: 8 in, 2 out]
          }
          frame "Go to Maint Tab" {
            n341 = call <vilib>:"Module.Window, Q Task.vi"("Action"=Window.Task,_Action."Show Maint Tab(Bool)", "Q In"=w731) -> ()  [unwired: 8 in, 2 out]
          }
        }
      }
      event User Event {
        n342 = event-data() -> ()  [unwired: 1 in, 5 out]
      }
      event "Clear Error": Value Change {
        n343 = event-data() -> ()  [unwired: 1 in, 6 out]
        n344 = call "Error.Clear.vi"("Q In"=w733) -> ()  [unwired: 9 in, 2 out]
      }
      event "Alias": Value Change {
        n345 = event-data() -> ()  [unwired: 1 in, 6 out]
        n346 = call <vilib>:"Q.Enqueue Task.vi"("Task Name"="Set Alias" ("Name"), "Q In"=w734) -> ()  [unwired: 8 in, 2 out]
      }
      event "Get ID": Value Change {
        n347 = event-data() -> ()  [unwired: 1 in, 6 out]
        n348 = call <vilib>:"Q.Enqueue Task.vi"("Task Name"="PS - Get ID" ("Name"), "Q In"=w736) -> ()  [unwired: 8 in, 2 out]
      }
      event "Toggle Sim": Value Change {
        n349 = event-data() -> ()  [unwired: 1 in, 6 out]
        n350 = call <vilib>:"Q.Enqueue Task.vi"("Task Name"="Simulate - Toggle" ("Name"), "Q In"=w738) -> ()  [unwired: 8 in, 2 out]
      }
      event "Read Current": Value Change {
        n351 = event-data() -> ()  [unwired: 1 in, 6 out]
        n352 = local write "Continuous Read"(FALSE ("Continuous Read")) -> ()
        n353 = call <vilib>:"Q.Enqueue Task.vi"("Task Name"="PS - Get Current", "Q In"=w741) -> ()  [unwired: 8 in, 2 out]
      }
      event "PS - Set Output ON", "PS - Set Output OFF": Value Change {
        n354 = event-data() -> ()  [unwired: 1 in, 6 out]
        n355 = To Variant(anything="PS - Set Output ON") -> (Variant=w744:variant)
        n356 = call <vilib>:"Q.Enqueue Task.vi"("Data1"=w744, "Task Name"="PS - Set Output", "Q In"=w745) -> ()  [unwired: 7 in, 2 out]
      }
      event "Save Current to File": Value Change {
        n357 = event-data() -> ()  [unwired: 1 in, 6 out]
        n358 = call <vilib>:"Q.Enqueue Task.vi"("Task Name"="Save Current to File", "Q In"=w747) -> ()  [unwired: 8 in, 2 out]
      }
      event "Clear Current Graph": Value Change {
        n359 = event-data() -> ()  [unwired: 1 in, 6 out]
        n360 = call <vilib>:"Q.Enqueue Task.vi"("Task Name"="Current Graph - Clear" ("Name"), "Q In"=w749) -> ()  [unwired: 8 in, 2 out]
      }
      event Value Change {
        n361 = event-data() -> ()  [unwired: 1 in, 6 out]
        n362 = To Variant(anything="Logging Level") -> (Variant=w752:variant)
        n363 = call <vilib>:"Q.Enqueue Task.vi"("Data1"=w752, "Task Name"="Set Logging Level", "Q In"=w754) -> ()  [unwired: 7 in, 2 out]
      }
      event "Continuous Read": Value Change {
        n364 = event-data() -> ("NewVal"=w755:bool)  [unwired: 1 in, 5 out]
        n365 = case shown="True" w755 {
          tunnel: w756 -> [_ w759]
          frame False {
          }
          frame True {
            n366 = call <vilib>:"Q.Enqueue Task.vi"("Task Name"="Current Graph - Clear" ("Name"), "Q In"=w759) -> ("Q Out"=w757:refnum<queue>)  [unwired: 8 in, 1 out]
            n367 = call <vilib>:"Q.Enqueue Task.vi"("Task Name"="PS - Get Current" ("Name"), "Q In"=w757) -> ()  [unwired: 8 in, 2 out]
          }
        }
      }
    }
  }
